vi "NEW数据采集传输系统.vi"() -> ()   [LabVIEW 2016, in "数据传输系统-04.lvlib"]
uses:
  <vilib>/Utility/miscctls.llb/LVPointTypeDef.ctl
  <vilib>/picture/picture.llb/imagedata.ctl
  <vilib>/Utility/config.llb/NI_LVConfig.lvlib
  update/update.lvlib
panel:
  in  "query":bool caption="返回"
  in  "每日自动重发":bool
  out "ADCP流程":string
  out "循环运行次数":i32
  out "上传动作":string
  out "在线ADCP分层数据时间":string
  out "海流计数据时间":string
  out "海流计流程":string
  in  "调试":u16(ring) items=["实时小时数据", "2086上传", "剖面多参数"]
  out "队列数量":u32
  out "数据查询指令":string
  out "2086上传":bool caption="2086"
  out "小时数据发送次数":i32
  out "选择发送的参数":string
  out "数值":i32
  in  "串口透传":bool
  in  "共享MN":bool
  out "剖面数据补发":bool
  out "日志信息补发":bool
  out "数据补发":bool
  in  "自动更新":bool
  in  "数据补传":bool caption="确定"
  out "数据库打开失败次数":dbl
  out "与工控通信指示灯":bool caption="与工控通信"
  out "判断数据反馈":enum16{"非严格判断", "严格判断", "不判断"}(ring)
  in  "暂停上传":bool
  in  "配置表":bool caption="确定"
  in  "updateconfiguration":T1={"主机"="27.154.58.30", "用户"="update", "密码"="std23506", "远程路径"="数据传输系统\\平台数据传输系统.exe", "下载文件名"="平台数据传输系统.exe", "软件版本"=""}
  out "标题显示":string
  in  "更新":bool
  in  "系统编码选择框":string(combo)="地表水质量监测"
  out "数据发送通道":enum16{"TCP", "VISA"}(ring)
  in  "baud rate":u32=9600 caption="波特率"
  in  "VISA resource name":refnum<visa-resource-name> caption="VISA资源名称"
  in  "实时数据发送时间间隔/min":i32=1
  in  "数据组合发送":bool
  in  "2011发送":bool
  out "数据发送协议":enum16{"2005-212协议", "2017-212协议"}(ring)=enum."2017-212协议"
  in  "重发时间":T2(ring)
  in  "重发日期":T3(ring)
  in  "开机启动":bool
  in  "每周自动重发":bool=TRUE
  in  "确定":bool
  in  "返回":bool
  in  "PW":string
  in  "MN":string
  in  "PORT":string
  in  "IP":string
  in  "站点设备":string
  in  "站点名称":string
  out "设置超时时间/min":i32=1
  out "状态信息":T4={"1st Error to Convert "=63, "步骤 "=enum."发送数据", "元素"="实时数据", "TCP服务端掉线计数"=0, "TCP掉线时间节点"="2019/05/08 15:24:17"} {"1st Error to Convert" items=["无错误", "参数错误", "内存已满", "超出区域", "文件结束", "文件已打开", "一般文件IO错误", "未找到文件", "文件权限错误", "磁盘已满", "路径副本", "打开过多文件", "未启用", "未找到资源文件", "无法添加资源", "未找到资源", "未找到图像", "图像内存错误", "画笔不存在", "配置错误类型", "配置未找到解析段", "配置解析错误", "配置内存错误", "错误外部代码格式", "错误外部代码偏移量", "外部代码不存在", "空窗口", "销毁窗口错误", "空菜单", "打印已中止", "错误打印记录", "打印驱动程序错误", "打印时窗口错误", "打印时内存错误", "打印对话框错误", "一般打印错误", "无效设备引用句柄", "设备未找到", "设备参数错误", "设备单位错误", "无法打开设备", "设备调用已中止", "一般错误", "用户已取消", "对象ID过低", "对象ID过高", "对象不在堆中", "未知的堆", "错误DefProc ID", "DefProc不在表格中", "范围外信息", "空方法", "未知信息", "不支持管理器调用", "错误地址", "连接过程中", "连接超时", "连接过程中", "不支持网络属性", "网络错误", "正在使用的地址", "系统缺少内存", "连接已中止", "连接已拒绝", "连接未建立", "连接已建立", "连接已关闭", "初始化错误（交互应用程序管理器）", "错误事件发生", "等待无约束事件发生处理程序", "事件发生队列溢出", "错误路径", "未发出信号量", "未识别类型（交互应用程序管理器）"]}
  out "数据接收超时指示灯":bool caption="数据接收超时"
  out "空闲时间/s":string
  out "系统时间":string
  out "实时小时数据上传":bool caption="实时小时数据"
  out "系统状态改变":bool
  out "软件版本":string
  out "掉线指示":bool
  out "核查数据上传":bool caption="核查数据"
  out "配置信息":T5
  in  "参数配置":bool
  out "反控数据发送":bool caption="反控数据"
  out "读取报文显示":string
  out "发送报文显示":string
  out "心跳包":bool
  out "通信状态":bool
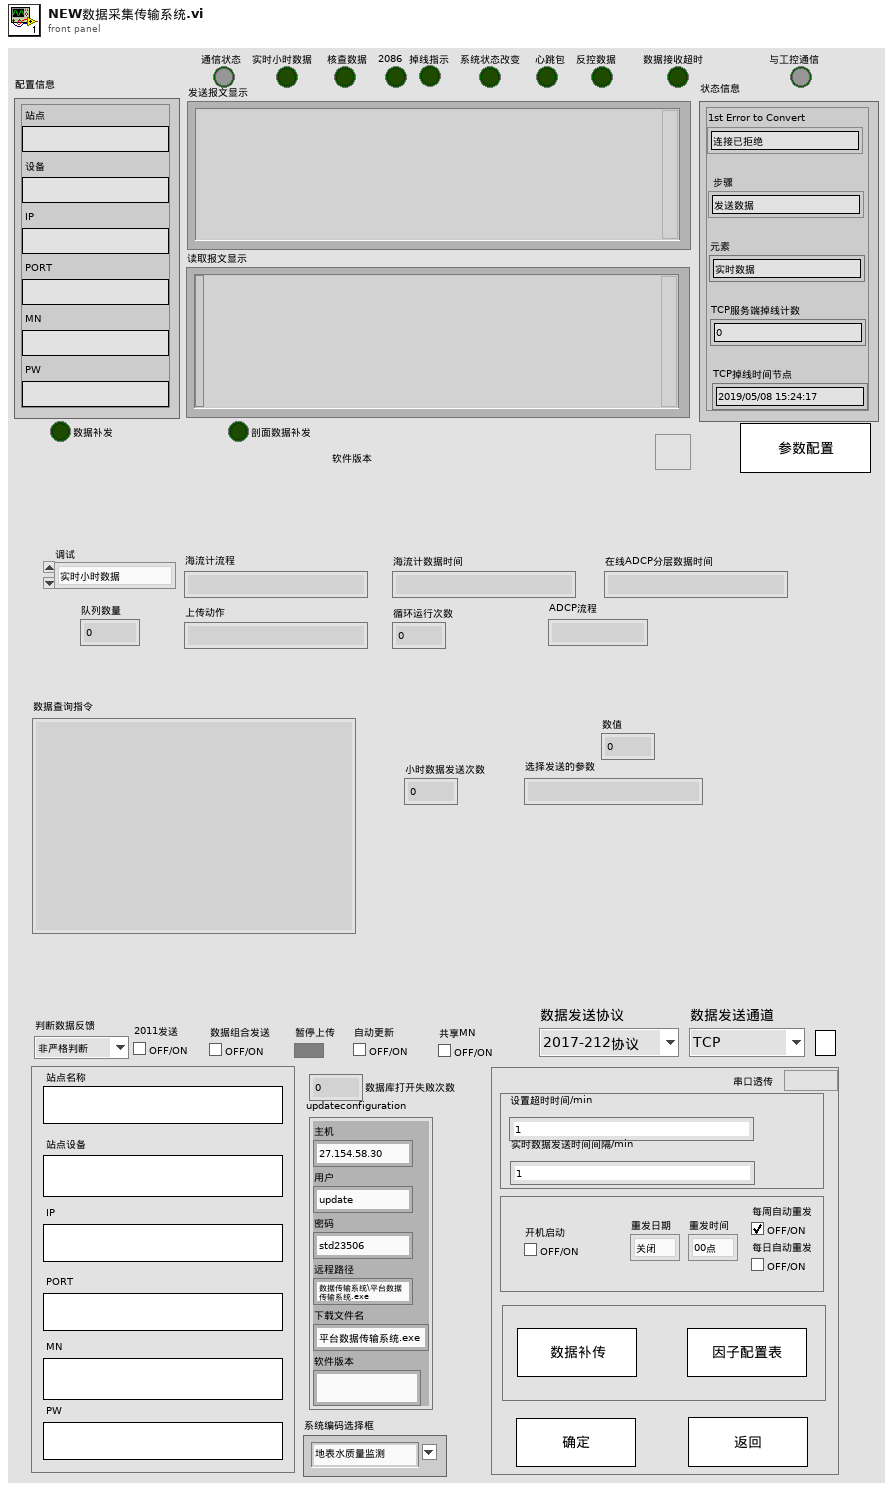
[diagram p1: front panel]
types:
  T1 = cluster{"主机":string, "用户":string, "密码":string, "远程路径":string, "下载文件名":string, "软件版本":string}
  T2 = enum16{"00点", "01点", "02点", "03点", "04点", "05点", "06点", "07点", "08点", "09点", "10点", "11点", "12点", "13点", "14点", "15点", "16点", "17点", "18点", "19点", "20点", "21点", "22点", "23点"}
  T3 = enum16{"关闭", "星期日", "星期一", "星期二", "星期三", "星期四", "星期五", "星期六"}
  T4 = cluster{"1st Error to Convert ":i32, "步骤 ":enum16{"打开连接", "发送数据", "读取数据", "数据处理", "关闭连接"}, "元素":string, "TCP服务端掉线计数":i32, "TCP掉线时间节点":string}
  T5 = cluster{"站点":string, "设备":string, "IP":string, "PORT":string, "MN":string, "PW":string}
  T6 = typedef "imagedata.ctl" = cluster{"image type":i32, "image depth":i32, "image":u8[], "mask":u8[], "colors":u32[], "Rectangle":cluster{"left":i16, "top":i16, "right":i16, "bottom":i16}}
  T7 = typedef "LVPointTypeDef.ctl" = cluster{"Horizontal":i16, "Vertical":i16}
  T8 = cluster{"setini":string, "sysini":string, "hechaini":string, "actualwrite":string, "actualread":string, "datasent":string, "反控命令信息队列":string, "反控与仪器交互":string}
  T9 = cluster{"配置表格[0]":string, "配置表格[1]":string, "配置表格[2]":string, "配置表格[3]":string, "配置表格[4]":string, "配置表格[5]":string, "配置表格[6]":string, "配置表格[7]":string, "配置表格[8]":string, "配置表格[9]":string, "配置表格[10]":string, "配置表格[11]":string, "配置表格[12]":string, "配置表格[13]":string, "配置表格[14]":string, "配置表格[15]":string, "配置表格[16]":string, "配置表格[17]":string, "配置表格[18]":string, "配置表格[19]":string, "配置表格[20]":string, "配置表格[21]":string, "配置表格[22]":string, "配置表格[23]":string, "配置表格[24]":string, "配置表格[25]":string, "配置表格[26]":string, "配置表格[27]":string, "配置表格[28]":string, "配置表格[29]":string, "配置表格[30]":string, "配置表格[31]":string, "配置表格[32]":string, "配置表格[33]":string, "配置表格[34]":string, "配置表格[35]":string, "配置表格[36]":string, "配置表格[37]":string, "配置表格[38]":string, "配置表格[39]":string, "配置表格[40]":string, "配置表格[41]":string, "配置表格[42]":string, "配置表格[43]":string, "配置表格[44]":string, "配置表格[45]":string, "配置表格[46]":string, "配置表格[47]":string, "配置表格[48]":string, "配置表格[49]":string, "配置表格[50]":string, "配置表格[51]":string, "配置表格[52]":string, "配置表格[53]":string, "配置表格[54]":string, "配置表格[55]":string, "配置表格[56]":string, "配置表格[57]":string, "配置表格[58]":string, "配置表格[59]":string, "配置表格[60]":string, "配置表格[61]":string, "配置表格[62]":string, "配置表格[63]":string, "配置表格[64]":string, "配置表格[65]":string, "配置表格[66]":string, "配置表格[67]":string, "配置表格[68]":string, "配置表格[69]":string, "配置表格[70]":string, "配置表格[71]":string, "配置表格[72]":string, "配置表格[73]":string, "配置表格[74]":string, "配置表格[75]":string}
  T10 = cluster{"[0]":dbl, "[1]":dbl, "[2]":dbl, "[3]":dbl, "[4]":dbl, "[5]":dbl, "[6]":dbl, "[7]":dbl, "[8]":dbl, "[9]":dbl, "[10]":dbl, "[11]":dbl, "[12]":dbl, "[13]":dbl, "[14]":dbl, "[15]":dbl, "[16]":dbl, "[17]":dbl, "[18]":dbl, "[19]":dbl, "[20]":dbl, "[21]":dbl, "[22]":dbl, "[23]":dbl, "[24]":dbl, "[25]":dbl, "[26]":dbl, "[27]":dbl, "[28]":dbl, "[29]":dbl, "[30]":dbl, "[31]":dbl, "[32]":dbl, "[33]":dbl, "[34]":dbl, "[35]":dbl, "[36]":dbl, "[37]":dbl, "[38]":dbl, "[39]":dbl, "[40]":dbl, "[41]":dbl, "[42]":dbl, "[43]":dbl, "[44]":dbl, "[45]":dbl, "[46]":dbl, "[47]":dbl, "[48]":dbl, "[49]":dbl, "[50]":dbl, "[51]":dbl, "[52]":dbl, "[53]":dbl, "[54]":dbl, "[55]":dbl, "[56]":dbl, "[57]":dbl, "[58]":dbl, "[59]":dbl, "[60]":dbl, "[61]":dbl, "[62]":dbl, "[63]":dbl, "[64]":dbl, "[65]":dbl, "[66]":dbl, "[67]":dbl, "[68]":dbl, "[69]":dbl, "[70]":dbl, "[71]":dbl, "[72]":dbl, "[73]":dbl, "[74]":dbl, "[75]":dbl}
  T11 = cluster{"时间标识":timestamp, "设备":string, "日志信息":string, "流程参数":string}
  T12 = typedef "NI_LVConfig.lvlib/Config Data RefNum.ctl" = refnum<k1>
  T13 = cluster{"[0]":bool, "[1]":bool, "[2]":bool, "[3]":bool, "[4]":bool, "[5]":bool, "[6]":bool, "[7]":bool, "[8]":bool, "[9]":bool, "[10]":bool, "[11]":bool, "[12]":bool, "[13]":bool, "[14]":bool, "[15]":bool, "[16]":bool, "[17]":bool, "[18]":bool, "[19]":bool, "[20]":bool, "[21]":bool, "[22]":bool, "[23]":bool, "[24]":bool, "[25]":bool, "[26]":bool, "[27]":bool, "[28]":bool, "[29]":bool, "[30]":bool, "[31]":bool, "[32]":bool, "[33]":bool, "[34]":bool, "[35]":bool, "[36]":bool, "[37]":bool, "[38]":bool, "[39]":bool, "[40]":bool, "[41]":bool, "[42]":bool, "[43]":bool, "[44]":bool, "[45]":bool, "[46]":bool, "[47]":bool, "[48]":bool, "[49]":bool, "[50]":bool, "[51]":bool, "[52]":bool, "[53]":bool, "[54]":bool, "[55]":bool, "[56]":bool, "[57]":bool, "[58]":bool, "[59]":bool, "[60]":bool, "[61]":bool, "[62]":bool, "[63]":bool, "[64]":bool, "[65]":bool, "[66]":bool, "[67]":bool, "[68]":bool, "[69]":bool, "[70]":bool, "[71]":bool, "[72]":bool, "[73]":bool, "[74]":bool, "[75]":bool}
  T14 = cluster{"time1":string, "time2":string, "time3":string, "time4":string, "time5":string, "time6":string, "time7":string, "time8":string, "time9":string, "time10":string, "time11":string, "time12":string, "time13":string, "time14":string, "time15":string, "time16":string, "time17":string, "time18":string, "time19":string, "time20":string, "time21":string, "time22":string, "time23":string, "time24":string, "time25":string, "time26":string, "time27":string, "time28":string, "time29":string, "time30":string, "time31":string, "time32":string, "time33":string, "time34":string, "time35":string, "time36":string, "time37":string, "time38":string, "time39":string, "time40":string, "time41":string, "time42":string, "time43":string, "time44":string, "time45":string, "time46":string, "time47":string, "time48":string, "time49":string, "time50":string, "time51":string, "time52":string, "time53":string, "time54":string, "time55":string, "time56":string, "time57":string, "time58":string, "time59":string, "time60":string, "time61":string, "time62":string, "time63":string, "time64":string, "time65":string, "time66":string, "time67":string, "time68":string, "time69":string, "time70":string, "time71":string, "time72":string, "time73":string, "time74":string, "time75":string, "time76":string}
  T15 = cluster{"[0]":string, "[1]":string, "[2]":string, "[3]":string, "[4]":string, "[5]":string, "[6]":string, "[7]":string}
  T16 = cluster{"[0]":string, "[1]":string, "[2]":string, "[3]":string, "[4]":string, "[5]":string, "[6]":string, "[7]":string, "[8]":string, "[9]":string, "[10]":string, "[11]":string, "[12]":string, "[13]":string, "[14]":string}
  T17 = cluster{"[0]":string, "[1]":string, "[2]":string, "[3]":string, "[4]":string, "[5]":string, "[6]":string}
  T18 = cluster{"[0]":string, "[1]":string, "[2]":string, "[3]":string, "[4]":string, "[5]":string, "[6]":string, "[7]":string, "[8]":string, "[9]":string, "[10]":string, "[11]":string, "[12]":string, "[13]":string, "[14]":string, "[15]":string, "[16]":string, "[17]":string}
  T19 = cluster{"[0]":string, "[1]":string, "[2]":string, "[3]":string, "[4]":string, "[5]":string, "[6]":string, "[7]":string, "[8]":string, "[9]":string}
  T20 = cluster{"[0]":string, "[1]":string, "[2]":string, "[3]":string, "[4]":string, "[5]":string, "[6]":string, "[7]":string, "[8]":string, "[9]":string, "[10]":string, "[11]":string, "[12]":string, "[13]":string, "[14]":string, "[15]":string, "[16]":string, "[17]":string, "[18]":string, "[19]":string, "[20]":string, "[21]":string, "[22]":string, "[23]":string, "[24]":string, "[25]":string, "[26]":string, "[27]":string, "[28]":string, "[29]":string, "[30]":string, "[31]":string, "[32]":string, "[33]":string, "[34]":string, "[35]":string, "[36]":string, "[37]":string, "[38]":string, "[39]":string, "[40]":string, "[41]":string, "[42]":string, "[43]":string, "[44]":string, "[45]":string, "[46]":string, "[47]":string, "[48]":string, "[49]":string, "[50]":string, "[51]":string, "[52]":string, "[53]":string, "[54]":string, "[55]":string, "[56]":string, "[57]":string, "[58]":string, "[59]":string, "[60]":string, "[61]":string, "[62]":string, "[63]":string, "[64]":string, "[65]":string, "[66]":string, "[67]":string, "[68]":string, "[69]":string, "[70]":string, "[71]":string, "[72]":string, "[73]":string, "[74]":string, "[75]":string}
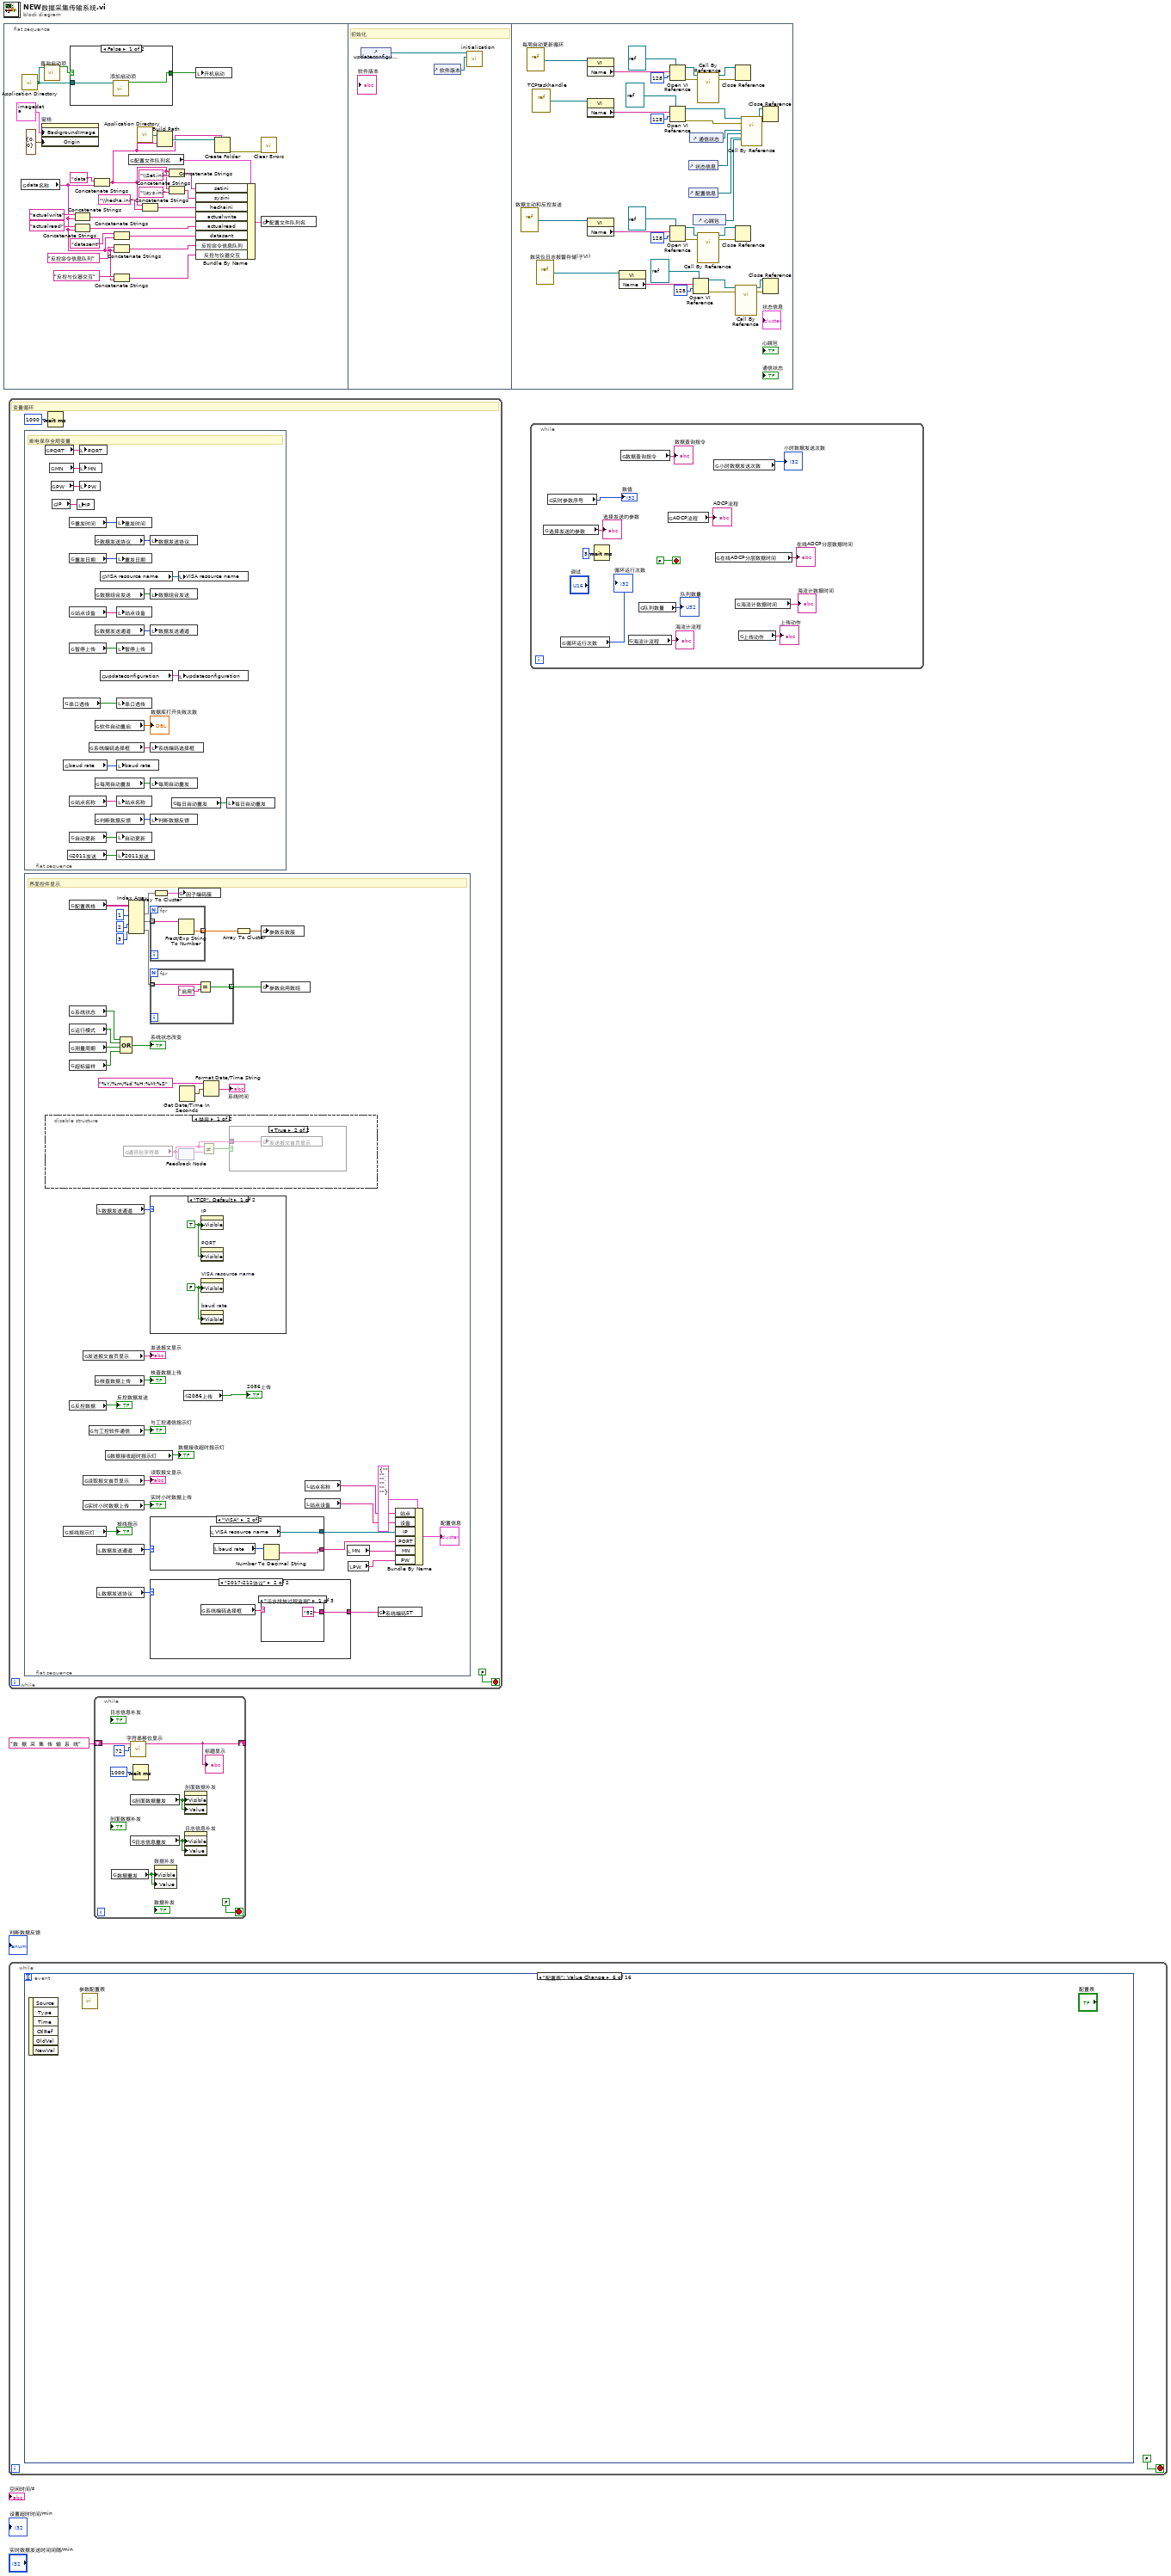
[diagram p0: block diagram]
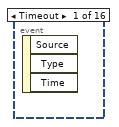
[diagram p2: hidden frame]
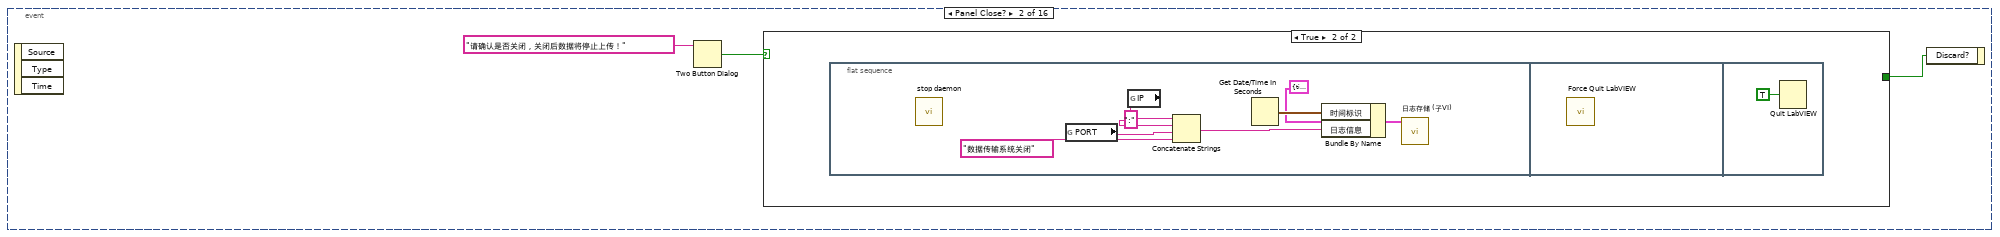
[diagram p3: hidden frame]
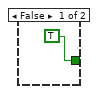
[diagram p4: hidden frame]
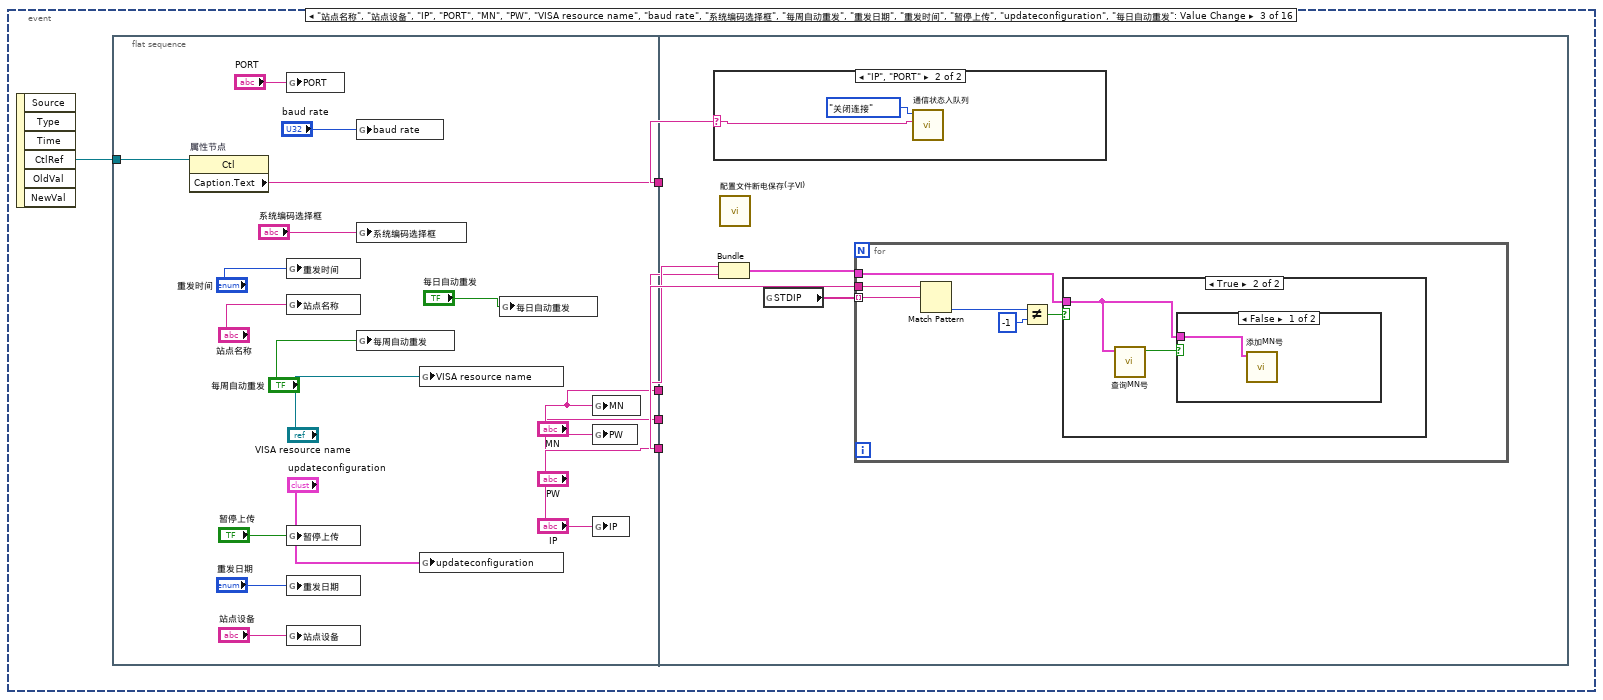
[diagram p5: hidden frame]
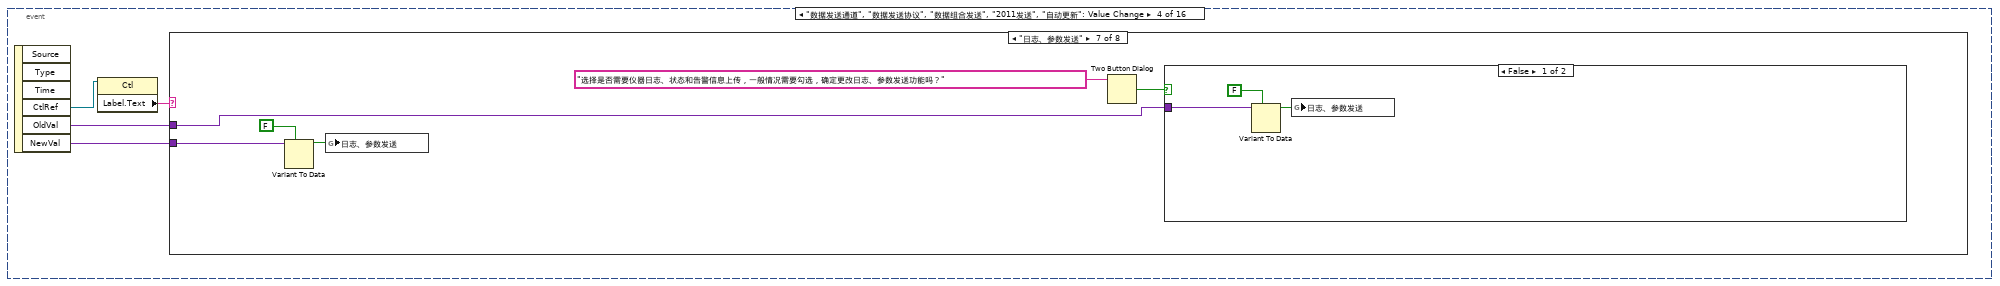
[diagram p9: hidden frame]
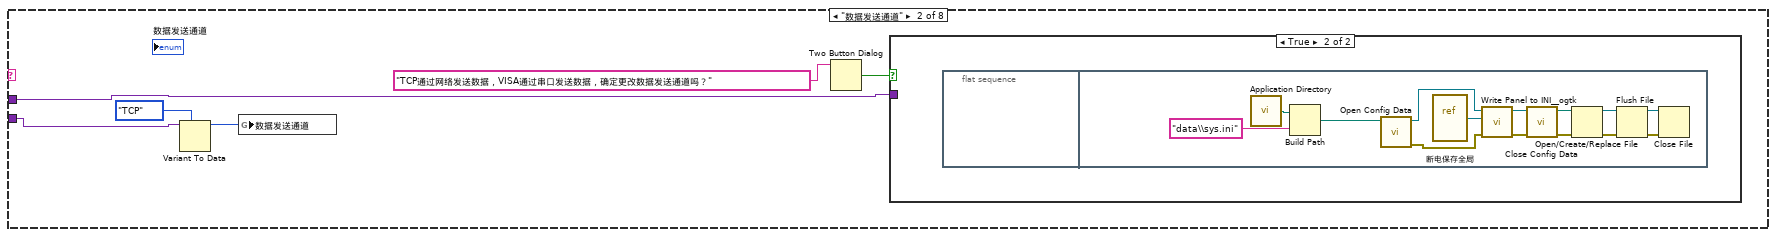
[diagram p11: hidden frame]
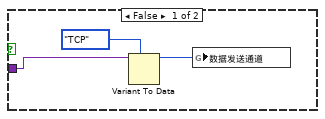
[diagram p12: hidden frame]
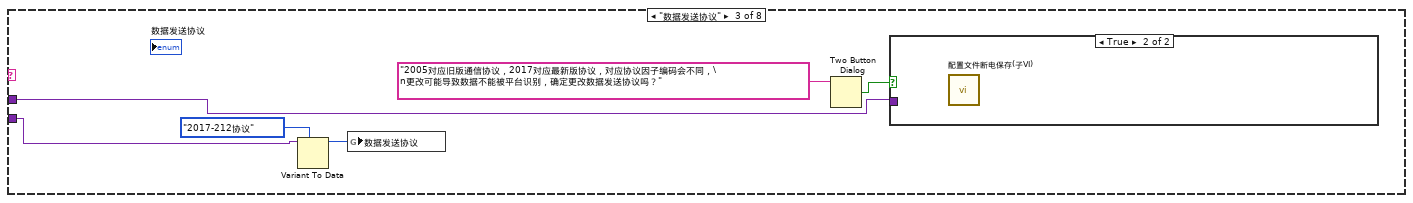
[diagram p13: hidden frame]
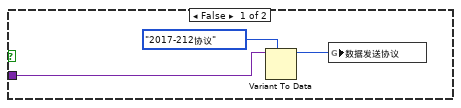
[diagram p14: hidden frame]
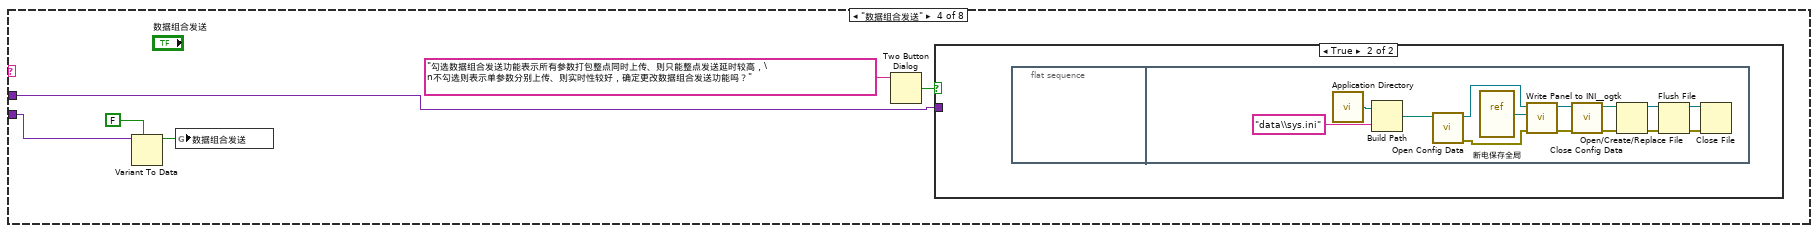
[diagram p15: hidden frame]
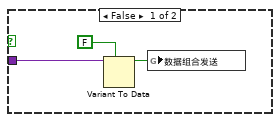
[diagram p16: hidden frame]
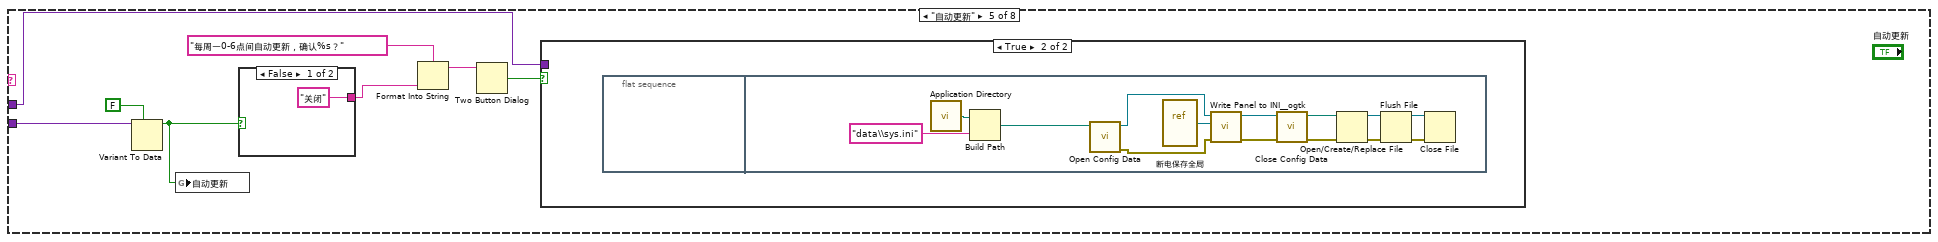
[diagram p17: hidden frame]
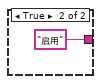
[diagram p18: hidden frame]
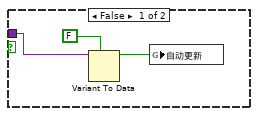
[diagram p19: hidden frame]
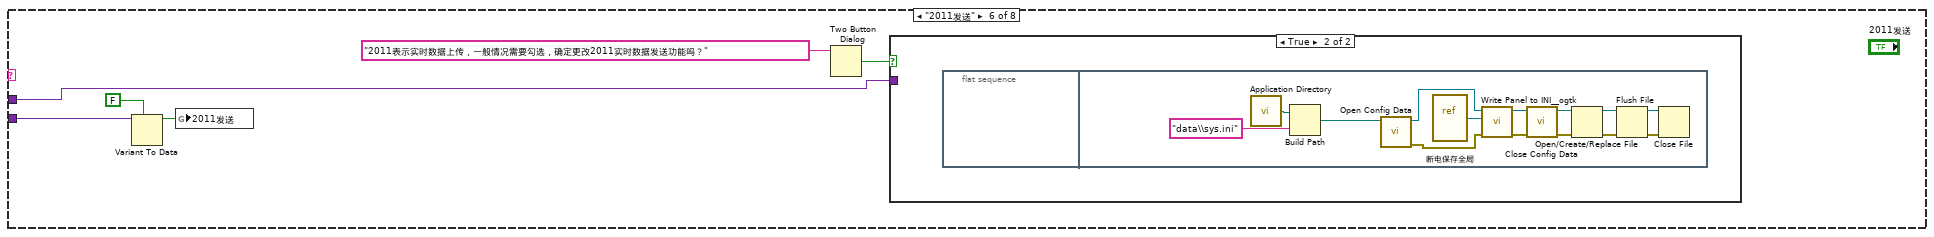
[diagram p20: hidden frame]
diagram:
  n1 = flat-sequence {
    frame #0 {
      n2 = global read "断电保存全局.vi" "data名称"() -> (w3:string)
      n3 = call <vilib>:"Application Directory.vi"() -> ("Application Directory"=w8:path)
      n4 = property on="窗格" class="Pane"("BackgroundImage"=T6 {"image type"=0, "image depth"=24, "image"=array[12288000 elements], "mask"=[], "colors"=[], "Rectangle"={"left"=0, "top"=0, "right"=2560, "bottom"=1600}} ("image data"), "Origin"=T7 {"Horizontal"=0, "Vertical"=0} ("原点")) -> ()  [unwired: 2 in, 2 out]
      n5 = call "查询启动项.vi"("启动文件路径"=w8) -> ("包含启动项"=w7:bool)  [unwired: 9 in, 1 out]
      n6 = case shown="False" w7 {
        selector: w7 -> [_ w33]
        tunnel: w8 -> [w32 _]
        tunnel: [w31 w33] -> w6
        frame False {
          n7 = call "添加启动项.vi"("启动文件路径"=w32) -> ("添加成功标记"=w31:bool)  [unwired: 9 in, 1 out]
        }
        frame True {
        }
      }
      n8 = Concatenate Strings("actualwrite" ("名称（未命名）"), w3) -> (w18:string)
      n9 = Concatenate Strings("actualread" ("名称（未命名）"), w3) -> (w16:string)
      n10 = Concatenate Strings("data" ("对话框窗口（创建文件夹）"), w3) -> (w23:string)
      n11 = Concatenate Strings("datasent" ("名称（未命名）"), w3) -> (w14:string)
      n12 = Concatenate Strings("反控命令信息队列" ("名称（未命名）"), w3) -> (w10:string)
      n13 = Concatenate Strings("反控与仪器交互" ("名称（未命名）"), w3) -> (w11:string)
      n14 = global read "全局1.vi" "配置文件队列名"() -> (w4:T8)
      n15 = call <vilib>:"Application Directory.vi"() -> ("Application Directory"=w29:path)
      n16 = Concatenate Strings(w23, "\\hecha.ini" ("名称或相对路径")) -> (w21:string)
      n17 = Build Path(base path=w29, name or relative path=w23) -> (appended path=w28:path)
      n18 = Concatenate Strings(w23, "\\Set.ini" ("名称或相对路径")) -> (w25:string)
      n19 = Concatenate Strings(w23, "\\sys.ini" ("名称或相对路径")) -> (w22:string)
      n20 = local write "开机启动"(w6) -> ()
      n21 = Bundle By Name(cluster=w4, "setini"=w25, "sysini"=w22, "hechaini"=w21, "actualwrite"=w18, "actualread"=w16, "datasent"=w14, "反控命令信息队列"=w10, "反控与仪器交互"=w11) -> (w2:T8)
      n22 = Create Folder(prompt (Create Folder)=w23, path (use dialog)=w28) -> (error out=w27:errorcluster)  [unwired: 1 in, 2 out]
      n23 = call <vilib>:"Clear Errors.vi"("error in (no error)"=w27) -> ()  [unwired: 5 in, 2 out]
      n24 = global write "全局1.vi" "配置文件队列名"(w2) -> ()
    }
    frame #1 {
      # "初始化"
      n25 = control-ref of="updateconfiguration"() -> (w35:refnum<vi>)
      n26 = control-ref of="软件版本"() -> (w34:refnum<vi>)
      n27 = call "initialization.vi"("软件版本"=w34, "updateconfiguration"=w35) -> ()  [unwired: 9 in]
    }
    frame #2 {
      n28 = vi-ref "数据主动和反控发送.vi"() -> (w36:refnum<vi>)
      n29 = vi-ref "每周自动更新循环.vi"() -> (w56:refnum<vi>)
      n30 = vi-ref "TCPtaskhandle.vi"() -> (w41:refnum<vi>)
      n31 = vi-ref "数采仪日志报警存储(子VI).vi"() -> (w64:refnum<vi>)
      n32 = property class="VI"(reference=w56) -> ("Name"=w49:string)  [unwired: 1 in, 2 out]
      n33 = property class="VI"(reference=w41) -> ("Name"=w48:string)  [unwired: 1 in, 2 out]
      n34 = property class="VI"(reference=w36) -> ("Name"=w63:string)  [unwired: 1 in, 2 out]
      n35 = property class="VI"(reference=w64) -> ("Name"=w71:string)  [unwired: 1 in, 2 out]
      n36 = Open VI Reference(type specifier VI Refnum (for type only)=refnum<vi> refnum, vi path=w49, options=128 ("选项")) -> (vi reference=w51:refnum<vi>, error out=w53:errorcluster)  [unwired: 3 in]
      n37 = Open VI Reference(type specifier VI Refnum (for type only)=refnum<vi> refnum, vi path=w48, options=128 ("选项")) -> (vi reference=w46:refnum<vi>, error out=w44:errorcluster)  [unwired: 3 in]
      n38 = Open VI Reference(type specifier VI Refnum (for type only)=refnum<vi> refnum, vi path=w63, options=128 ("选项")) -> (vi reference=w61:refnum<vi>, error out=w59:errorcluster)  [unwired: 3 in]
      n39 = control-ref of="状态信息"() -> (w39:refnum<vi>)
      n40 = control-ref of="配置信息"() -> (w38:refnum<vi>)
      n41 = control-ref of="通信状态"() -> (w40:refnum<vi>)
      n42 = control-ref of="心跳包"() -> (w37:refnum<vi>)
      n43 = Open VI Reference(type specifier VI Refnum (for type only)=refnum<vi> refnum, vi path=w71, options=128 ("选项")) -> (vi reference=w69:refnum<vi>, error out=w67:errorcluster)  [unwired: 3 in]
      n44 = call-by-ref "?"(reference=w51, error in=w53) -> (reference out=w55:refnum<vi>, error out=w54:errorcluster)  [unwired: 12 in]
      n45 = call-by-ref "?"(reference=w61, error in=w59) -> (reference out=w57:refnum<vi>, error out=w58:errorcluster)  [unwired: 12 in]
      n46 = Close Reference(reference=w55, error in (no error)=w54) -> ()  [unwired: 1 out]
      n47 = Close Reference(reference=w57, error in (no error)=w58) -> ()  [unwired: 1 out]
      n48 = call-by-ref "?"(reference=w69, error in=w67) -> (reference out=w65:refnum<vi>, error out=w66:errorcluster)  [unwired: 12 in]
      n49 = call-by-ref "?"(reference=w46, error in=w44, "心跳包"=w37, "配置信息"=w38, "状态信息"=w39, "通信状态"=w40) -> (reference out=w42:refnum<vi>, error out=w43:errorcluster)  [unwired: 8 in]
      n50 = Close Reference(reference=w42, error in (no error)=w43) -> ()  [unwired: 1 out]
      n51 = Close Reference(reference=w65, error in (no error)=w66) -> ()  [unwired: 1 out]
    }
  }
  n52 = while {
    stop <- FALSE stop-if-true
    # "变量循环"
    n53 = flat-sequence {
      frame #0 {
        # "断电保存全局变量"
        n54 = global read "断电保存全局.vi" "PORT"() -> (w161:string)
        n55 = global read "断电保存全局.vi" "MN"() -> (w160:string)
        n56 = global read "断电保存全局.vi" "PW"() -> (w159:string)
        n57 = global read "断电保存全局.vi" "IP"() -> (w162:string)
        n58 = global read "断电保存全局.vi" "串口透传"() -> (w143:bool)
        n59 = global read "断电保存全局.vi" "baud rate"() -> (w157:u32)
        n60 = global read "断电保存全局.vi" "2011发送"() -> (w153:bool)
        n61 = global read "断电保存全局.vi" "重发时间"() -> (w148:T2)
        n62 = global read "断电保存全局.vi" "重发日期"() -> (w155:T3)
        n63 = global read "断电保存全局.vi" "站点设备"() -> (w163:string)
        n64 = global read "断电保存全局.vi" "暂停上传"() -> (w147:bool)
        n65 = global read "断电保存全局.vi" "站点名称"() -> (w164:string)
        n66 = global read "断电保存全局.vi" "自动更新"() -> (w145:bool)
        n67 = local write "IP"(w162) -> ()
        n68 = local write "PORT"(w161) -> ()
        n69 = local write "MN"(w160) -> ()
        n70 = local write "PW"(w159) -> ()
        n71 = global read "断电保存全局.vi" "系统编码选择框"() -> (w149:string)
        n72 = global read "断电保存全局.vi" "数据发送协议"() -> (w151:enum16{"2005-212协议", "2017-212协议"})
        n73 = global read "断电保存全局.vi" "数据组合发送"() -> (w152:bool)
        n74 = global read "断电保存全局.vi" "数据发送通道"() -> (w150:enum16{"TCP", "VISA"})
        n75 = global read "全局1.vi" "软件自动重启"() -> (→"数据库打开失败次数":dbl)
        n76 = global read "断电保存全局.vi" "每周自动重发"() -> (w156:bool)
        n77 = global read "断电保存全局.vi" "判断数据反馈"() -> (w154:enum16{"非严格判断", "严格判断", "不判断"})
        n78 = global read "断电保存全局.vi" "VISA resource name"() -> (w158:refnum<visa-resource-name>)
        n79 = global read "断电保存全局.vi" "updateconfiguration"() -> (w144:T1)
        n80 = local write "重发时间"(w148) -> ()
        n81 = local write "重发日期"(w155) -> ()
        n82 = local write "站点设备"(w163) -> ()
        n83 = local write "暂停上传"(w147) -> ()
        n84 = local write "串口透传"(w143) -> ()
        n85 = local write "baud rate"(w157) -> ()
        n86 = local write "站点名称"(w164) -> ()
        n87 = local write "自动更新"(w145) -> ()
        n88 = local write "2011发送"(w153) -> ()
        n89 = local write "数据发送协议"(w151) -> ()
        n90 = local write "数据组合发送"(w152) -> ()
        n91 = local write "数据发送通道"(w150) -> ()
        n92 = local write "系统编码选择框"(w149) -> ()
        n93 = local write "每周自动重发"(w156) -> ()
        n94 = local write "判断数据反馈"(w154) -> ()
        n95 = global read "断电保存全局.vi" "每日自动重发"() -> (w142:bool)
        n96 = local write "VISA resource name"(w158) -> ()
        n97 = local write "updateconfiguration"(w144) -> ()
        n98 = local write "每日自动重发"(w142) -> ()
      }
    }
    n99 = flat-sequence {
      frame #0 {
        # "界面控件显示"
        n100 = disable-structure shown="禁用" {
          frame Disabled {
            n101 = global read "全局1.vi" "通讯包字符串"() -> (w115:string)
            n102 = feedback #1(w115) -> (w116:string)
            n103 = feedback-in #1(w115) -> ()
            n104 = Not Equal?(x=w115, y=w116) -> (x != y?=w114:bool)
            n105 = case shown="True" w114 {
              tunnel: w115 -> [_ w117]
              frame False {
              }
              frame True {
                n106 = global write "全局1.vi" "发送报文首页显示"(w117) -> ()
              }
            }
          }
          frame Enabled {
          }
        }
        n107 = global read "全局 数据发送重叠.vi" "掉线指示灯"() -> (→"掉线指示":bool)
        n108 = global read "断电保存全局.vi" "配置表格"() -> (w85:string[][])
        n109 = global read "全局1.vi" "系统状态"() -> (w87:bool)
        n110 = global read "全局1.vi" "运行模式"() -> (w88:bool)
        n111 = global read "全局1.vi" "测量周期"() -> (w89:bool)
        n112 = global read "全局1.vi" "超标留样"() -> (w90:bool)
        n113 = global read "全局1.vi" "反控数据"() -> (→"反控数据发送":bool)
        n114 = global read "全局1.vi" "发送报文首页显示"() -> (→"发送报文显示":string)
        n115 = global read "全局1.vi" "读取报文首页显示"() -> (→"读取报文显示":string)
        n116 = global read "全局1.vi" "实时小时数据上传"() -> (→"实时小时数据上传":bool)
        n117 = global read "全局1.vi" "与工控软件通信"() -> (→"与工控通信指示灯":bool)
        n118 = global read "全局1.vi" "核查数据上传"() -> (→"核查数据上传":bool)
        n119 = local read "数据发送通道"() -> (w95:enum16{"TCP", "VISA"})
        n120 = local read "数据发送通道"() -> (w113:enum16{"TCP", "VISA"})
        n121 = local read "数据发送协议"() -> (w102:enum16{"2005-212协议", "2017-212协议"})
        n122 = global read "全局 数据发送重叠.vi" "数据接收超时指示灯"() -> (→"数据接收超时指示灯":bool)
        n123 = Compound Arithmetic op=OR ("复合运算")(w87, w88, w89, w90) -> (→"系统状态改变":bool)
        n124 = Index Array(array=w85, index (col) #1=1 ("禁用的索引 (列)"), index (col) #2=2 ("索引 (列)"), index (col) #3=3 ("索引 (列)")) -> (element #1=w83:string[], element #2=w77:string[], element #3=w79:string[])  [unwired: 3 in]
        n125 = for {
          tunnel: w77 -> [w119] mode=indexing
          tunnel: [w118] -> w76 mode=indexing
          n126 = Fract/Exp String To Number(string=w119) -> (number=w118:dbl)  [unwired: 3 in, 1 out]
        }
        n127 = for {
          tunnel: w79 -> [w122] mode=indexing
          tunnel: [w120] -> w78 mode=indexing
          n128 = Equal?(x=w122, y="启用") -> (x = y?=w120:bool)
        }
        n129 = case shown="\"TCP\", Default" w95 {
          frame "TCP", Default {
            w123 = TRUE ("可见")
            w124 = FALSE ("可见")
            n130 = property on="IP" class="Str"("Visible"=w123) -> ()  [unwired: 2 in, 2 out]
            n131 = property on="PORT" class="Str"("Visible"=w123) -> ()  [unwired: 2 in, 2 out]
            n132 = property on="VISA resource name" class="VISAName"("Visible"=w124) -> ()  [unwired: 2 in, 2 out]
            n133 = property on="baud rate" class="DigNum (strict)"("Visible"=w124) -> ()  [unwired: 2 in, 2 out]
          }
          frame "VISA" {
            w125 = FALSE ("可见")
            w126 = TRUE ("可见")
            n134 = property on="IP" class="Str"("Visible"=w125) -> ()  [unwired: 2 in, 2 out]
            n135 = property on="PORT" class="Str"("Visible"=w125) -> ()  [unwired: 2 in, 2 out]
            n136 = property on="VISA resource name" class="VISAName"("Visible"=w126) -> ()  [unwired: 2 in, 2 out]
            n137 = property on="baud rate" class="DigNum (strict)"("Visible"=w126) -> ()  [unwired: 2 in, 2 out]
          }
        }
        n138 = case shown="\"VISA\"" w113 {
          tunnel: [w138 w141] -> w110
          tunnel: [w137 w139] -> w107
          frame "TCP", Default {
            n139 = local read "PORT"() -> (w137:string)
            n140 = local read "IP"() -> (w138:string)
          }
          frame "VISA" {
            n141 = local read "VISA resource name"() -> (w141:refnum<visa-resource-name>)
            n142 = local read "baud rate"() -> (w140:u32)
            n143 = Number To Decimal String(number=w140) -> (decimal integer string=w139:string)  [unwired: 1 in]
          }
        }
        n144 = case shown="\"2017-212协议\"" w102 {
          tunnel: [w127 w132] -> w101
          frame "2005-212协议", Default {
            n145 = global read "断电保存全局.vi" "系统编码选择框"() -> (w128:string)
            n146 = case shown="\"地表水体污染源\"" w128 {
              tunnel: ["52" ("设备编码MN") "32" ("设备编码MN") "21" ("设备编码MN")] -> w127
              frame "污水排放过程监测" {
              }
              frame "地表水体污染源" {
              }
              frame "地表水质量监测", Default {
              }
            }
          }
          frame "2017-212协议" {
            n147 = global read "断电保存全局.vi" "系统编码选择框"() -> (w133:string)
            n148 = case shown="\"污水排放过程监测\"" w133 {
              tunnel: ["52" ("设备编码MN") "32" ("设备编码MN") "21" ("设备编码MN")] -> w132
              frame "污水排放过程监测" {
              }
              frame "地表水体污染源" {
              }
              frame "地表水质量监测", Default {
              }
            }
          }
        }
        n149 = Array To Cluster(array=w83) -> (cluster=w86:T9)
        n150 = global write "断电保存全局.vi" "因子编码簇"(w86) -> ()
        n151 = Get Date/Time In Seconds() -> (seconds since 1Jan1904=w103:timestamp)
        n152 = global read "全局1.vi" "2086上传"() -> (→"2086上传":bool)
        n153 = Format Date/Time String(time format string (%c)="%Y/%m/%d %H:%M:%S" ("时间格式字符串(%c)"), seconds (now)=w103) -> (date/time string=→"系统时间":string)  [unwired: 1 in]
        n154 = Array To Cluster(array=w76) -> (cluster=w80:T10)
        n155 = global write "断电保存全局.vi" "参数系数簇"(w80) -> ()
        n156 = global write "断电保存全局.vi" "参数启用数组"(w78) -> ()
        n157 = local read "站点名称"() -> (w109:string)
        n158 = local read "站点设备"() -> (w108:string)
        n159 = local read "MN"() -> (w106:string)
        n160 = local read "PW"() -> (w105:string)
        n161 = global write "全局1.vi" "系统编码ST"(w101) -> ()
        n162 = Bundle By Name(cluster=T5 {"站点"="", "设备"="", "IP"="", "PORT"="", "MN"="", "PW"=""} ("配置信息"), "站点"=w109, "设备"=w108, "IP"=w110, "PORT"=w107, "MN"=w106, "PW"=w105) -> (→"配置信息":T5)
      }
    }
    n163 = Wait (ms)(milliseconds to wait=u32 1000 ("等待时间（毫秒）")) -> ()  [unwired: 1 out]
  }
  n164 = while {
    stop <- FALSE stop-if-true
    n165 = event shown="[5] \"配置表\": Value Change" {
      selector: _ -> [_ _ _ _ _ _ _ _ _ _ _ _ _ _ _ _]
      dyn-events: _ -> [_ _ _ _ _ _ _ _ _ _ _ _ _ _ _ _]
      timeout: _ -> [_ _ _ _ _ _ _ _ _ _ _ _ _ _ _ _]
      event Timeout {
        n166 = event-data() -> ()  [unwired: 1 in, 3 out]
      }
      event Panel Close? {
        n167 = event-data() -> ()  [unwired: 1 in, 3 out]
        n168 = Two Button Dialog(message="请确认是否关闭，关闭后数据将停止上传！" ("消息")) -> (T button?=w167:bool)  [unwired: 2 in]
        n169 = case shown="True" w167 {
          tunnel: [TRUE _] -> w166
          frame False {
          }
          frame True {
            n170 = flat-sequence {
              frame #0 {
                n171 = call "stop daemon.vi"() -> ()  [unwired: 11 in, 1 out]
                n172 = global read "断电保存全局.vi" "PORT"() -> (w173:string)
                n173 = global read "断电保存全局.vi" "IP"() -> (w175:string)
                n174 = Concatenate Strings(w175, ":", w173, "数据传输系统关闭" ("日志信息")) -> (w171:string)
                n175 = Get Date/Time In Seconds() -> (seconds since 1Jan1904=w177:timestamp)
                n176 = Bundle By Name(cluster=T11 {"时间标识"=timestamp(0 s since 1904-01-01), "设备"="数采仪", "日志信息"="", "流程参数"=""} ("data in"), "时间标识"=w177, "日志信息"=w171) -> (w176:T11)
                n177 = call "日志存储 (子VI).vi"("data in"=w176) -> ()  [unwired: 11 in]
              }
              frame #1 {
                n178 = call "Force Quit LabVIEW.vi"() -> ()  [unwired: 10 in, 2 out]
              }
              frame #2 {
                n179 = Quit LabVIEW(quit? (T)=TRUE ("退出？(T)")) -> ()
              }
            }
          }
        }
        n180 = event-data("Discard?"=w166) -> ()  [unwired: 1 in, 1 out]
      }
      event "站点名称", "站点设备", "IP", "PORT", "MN", "PW", "VISA resource name", "baud rate", "系统编码选择框", "每周自动重发", "重发日期", "重发时间", "暂停上传", "updateconfiguration", "每日自动重发": Value Change {
        n181 = event-data() -> ("CtlRef"=w183:refnum<vi>)  [unwired: 1 in, 5 out]
        n182 = flat-sequence {
          tunnel: w183 -> [w185]
          tunnel: [w190] -> w182
          tunnel: ["IP"] -> w181
          tunnel: ["MN"] -> w180
          tunnel: ["PW"] -> w179
          tunnel: w182 -> [w206]
          tunnel: w181 -> [w204]
          tunnel: w180 -> [w203]
          tunnel: w179 -> [w202]
          frame #0 {
            n183 = property on="属性节点" class="Ctl"(reference=w185) -> ("Caption.Text"=w190:string)  [unwired: 1 in, 2 out]
            n184 = global write "断电保存全局.vi" "PORT"("PORT") -> ()
            n185 = global write "断电保存全局.vi" "重发时间"("重发时间") -> ()
            n186 = global write "断电保存全局.vi" "站点名称"("站点名称") -> ()
            n187 = global write "断电保存全局.vi" "暂停上传"("暂停上传") -> ()
            n188 = global write "断电保存全局.vi" "重发日期"("重发日期") -> ()
            n189 = global write "断电保存全局.vi" "站点设备"("站点设备") -> ()
            n190 = global write "断电保存全局.vi" "baud rate"("baud rate") -> ()
            n191 = global write "断电保存全局.vi" "系统编码选择框"("系统编码选择框") -> ()
            n192 = global write "断电保存全局.vi" "每周自动重发"("每周自动重发") -> ()
            n193 = global write "断电保存全局.vi" "VISA resource name"("VISA resource name") -> ()
            n194 = global write "断电保存全局.vi" "updateconfiguration"("updateconfiguration") -> ()
            n195 = global write "断电保存全局.vi" "每日自动重发"("每日自动重发") -> ()
            n196 = global write "断电保存全局.vi" "MN"("MN") -> ()
            n197 = global write "断电保存全局.vi" "PW"("PW") -> ()
            n198 = global write "断电保存全局.vi" "IP"("IP") -> ()
          }
          frame #1 {
            n199 = case shown="\"IP\", \"PORT\"" w206 {
              selector: w206 -> [_ w216]
              frame "假", Default {
              }
              frame "IP", "PORT" {
                n200 = call "通信状态入队列.vi"("发送报文"=w216, "枚举"=enum16{"打开连接", "发送数据", "读取数据", "数据处理", "关闭连接"}."关闭连接") -> ()  [unwired: 9 in, 1 out]
              }
            }
            n201 = Bundle("MN"=w203, "PW"=w202) -> (w201:cluster{"MN":string, "PW":string})  [unwired: 1 in]
            n202 = call "配置文件断电保存(子VI).vi"() -> ()  [unwired: 12 in]
            n203 = global read "断电保存全局.vi" "STDIP"() -> (w205:string[])
            n204 = for {
              tunnel: w205 -> [w212] mode=indexing
              tunnel: w204 -> [w211]
              tunnel: w201 -> [w207]
              n205 = Match Pattern(string=w211, regular expression=w212) -> (offset past match=w210:i32)  [unwired: 1 in, 3 out]
              n206 = Not Equal?(x=w210, y=-1) -> (x != y?=w208:bool)
              n207 = case shown="True" w208 {
                tunnel: w207 -> [_ w214]
                frame False {
                }
                frame True {
                  n208 = call "查询MN号.vi"("簇"=w214) -> ("包含启动项"=w213:bool)  [unwired: 9 in, 1 out]
                  n209 = case shown="False" w213 {
                    tunnel: w214 -> [w215 _]
                    frame False {
                      n210 = call "添加MN号.vi"("簇"=w215) -> ()  [unwired: 9 in, 2 out]
                    }
                    frame True {
                    }
                  }
                }
              }
            }
          }
        }
      }
      event "数据发送通道", "数据发送协议", "数据组合发送", "2011发送", "自动更新": Value Change {
        n211 = event-data() -> ("CtlRef"=w221:refnum<vi>, "OldVal"=w219:variant, "NewVal"=w218:variant)  [unwired: 1 in, 3 out]
        n212 = property class="Ctl"(reference=w221) -> ("Label.Text"=w220:string)  [unwired: 1 in, 2 out]
        n213 = case shown="\"日志、参数发送\"" w220 {
          tunnel: w219 -> [_ w225 w248 w257 w283 w307 w330 w351]
          tunnel: w218 -> [_ w222 w245 w254 w281 w304 w327 w350]
          frame "假", Default {
          }
          frame "数据发送通道" {
            n214 = Variant To Data(type=enum16{"TCP", "VISA"}."TCP" ("数据发送通道"), Variant=w222) -> (data=w223:enum16{"TCP", "VISA"})  [unwired: 1 in, 1 out]
            n215 = global write "断电保存全局.vi" "数据发送通道"(w223) -> ()
            n216 = Two Button Dialog(message="TCP通过网络发送数据，VISA通过串口发送数据，确定更改数据发送通道吗？" ("消息")) -> (T button?=w226:bool)  [unwired: 2 in]
            n217 = case shown="True" w226 {
              tunnel: w225 -> [w229 _]
              frame False {
                n218 = Variant To Data(type=enum16{"TCP", "VISA"}."TCP" ("数据发送通道"), Variant=w229) -> (data=w228:enum16{"TCP", "VISA"})  [unwired: 1 in, 1 out]
                n219 = global write "断电保存全局.vi" "数据发送通道"(w228) -> ()
              }
              frame True {
                n220 = flat-sequence {
                  frame #0 {
                  }
                  frame #1 {
                    n221 = call <vilib>:"Application Directory.vi"() -> ("Application Directory"=w231:path)
                    n222 = Build Path(base path=w231, name or relative path="data\\sys.ini" ("名称或相对路径")) -> (appended path=w233:path)
                    n223 = call <vilib>:"Open Config Data.vi"("configuration file path"=w233) -> ("error out"=w237:errorcluster, "refnum"=w234:T12)  [unwired: 8 in, 1 out]
                    n224 = vi-ref "断电保存全局.vi"() -> (w235:refnum<vi>)
                    n225 = call <userlib>:"Write Panel to INI__ogtk.vi"("error in (no error)"=w237, "VI ref"=w235, "refnum"=w234) -> ("error out"=w238:errorcluster, "refnum out"=w236:T12)  [unwired: 7 in]
                    n226 = call <vilib>:"Close Config Data.vi"("error in (no error)"=w238, "refnum"=w236) -> ("error out"=w243:errorcluster, "file path"=w244:path)  [unwired: 8 in]
                    n227 = Open/Create/Replace File(file path (use dialog)=w244, error in=w243) -> (refnum out=w240:refnum<file>, error out=w239:errorcluster)  [unwired: 4 in, 1 out]
                    n228 = Flush File(refnum=w240, error in=w239) -> (refnum out=w241:refnum<file>, error out=w242:errorcluster)
                    n229 = Close File(refnum=w241, error in=w242) -> ()  [unwired: 2 out]
                  }
                }
              }
            }
          }
          frame "数据发送协议" {
            n230 = Variant To Data(type=enum16{"2005-212协议", "2017-212协议"}."2017-212协议" ("数据"), Variant=w245) -> (data=w246:enum16{"2005-212协议", "2017-212协议"})  [unwired: 1 in, 1 out]
            n231 = global write "断电保存全局.vi" "数据发送协议"(w246) -> ()
            n232 = Two Button Dialog(message="2005对应旧版通信协议，2017对应最新版协议，对应协议因子编码会不同，\n更改可能导致数据不能被平台识别，确定更改数据发送协议吗？" ("消息")) -> (T button?=w249:bool)  [unwired: 2 in]
            n233 = case shown="True" w249 {
              tunnel: w248 -> [w253 _]
              frame False {
                n234 = Variant To Data(type=enum16{"2005-212协议", "2017-212协议"}."2017-212协议" ("数据"), Variant=w253) -> (data=w251:enum16{"2005-212协议", "2017-212协议"})  [unwired: 1 in, 1 out]
                n235 = global write "断电保存全局.vi" "数据发送协议"(w251) -> ()
              }
              frame True {
                n236 = call "配置文件断电保存(子VI).vi"() -> ()  [unwired: 12 in]
              }
            }
          }
          frame "数据组合发送" {
            n237 = Variant To Data(type=FALSE, Variant=w254) -> (data=w255:bool)  [unwired: 1 in, 1 out]
            n238 = global write "断电保存全局.vi" "数据组合发送"(w255) -> ()
            n239 = Two Button Dialog(message="勾选数据组合发送功能表示所有参数打包整点同时上传、则只能整点发送延时较高，\n不勾选则表示单参数分别上传、则实时性较好，确定更改数据组合发送功能吗？" ("消息")) -> (T button?=w258:bool)  [unwired: 2 in]
            n240 = case shown="True" w258 {
              tunnel: w257 -> [w261 _]
              frame False {
                n241 = Variant To Data(type=FALSE, Variant=w261) -> (data=w260:bool)  [unwired: 1 in, 1 out]
                n242 = global write "断电保存全局.vi" "数据组合发送"(w260) -> ()
              }
              frame True {
                n243 = flat-sequence {
                  frame #0 {
                  }
                  frame #1 {
                    n244 = call <vilib>:"Application Directory.vi"() -> ("Application Directory"=w263:path)
                    n245 = Build Path(base path=w263, name or relative path="data\\sys.ini" ("名称或相对路径")) -> (appended path=w265:path)
                    n246 = call <vilib>:"Open Config Data.vi"("configuration file path"=w265) -> ("error out"=w269:errorcluster, "refnum"=w266:T12)  [unwired: 8 in, 1 out]
                    n247 = vi-ref "断电保存全局.vi"() -> (w267:refnum<vi>)
                    n248 = call <userlib>:"Write Panel to INI__ogtk.vi"("error in (no error)"=w269, "VI ref"=w267, "refnum"=w266) -> ("error out"=w270:errorcluster, "refnum out"=w268:T12)  [unwired: 7 in]
                    n249 = call <vilib>:"Close Config Data.vi"("error in (no error)"=w270, "refnum"=w268) -> ("error out"=w275:errorcluster, "file path"=w276:path)  [unwired: 8 in]
                    n250 = Open/Create/Replace File(file path (use dialog)=w276, error in=w275) -> (refnum out=w272:refnum<file>, error out=w271:errorcluster)  [unwired: 4 in, 1 out]
                    n251 = Flush File(refnum=w272, error in=w271) -> (refnum out=w273:refnum<file>, error out=w274:errorcluster)
                    n252 = Close File(refnum=w273, error in=w274) -> ()  [unwired: 2 out]
                  }
                }
              }
            }
          }
          frame "自动更新" {
            n253 = Variant To Data(type=FALSE, Variant=w281) -> (data=w279:bool)  [unwired: 1 in, 1 out]
            n254 = global write "断电保存全局.vi" "自动更新"(w279) -> ()
            n255 = case shown="False" w279 {
              tunnel: ["关闭" "启用"] -> w278
              frame False {
              }
              frame True {
              }
            }
            n256 = Format Into String(format string="每周一0-6点间自动更新，确认%s？" ("消息"), w278) -> (resulting string=w277:string)  [unwired: 2 in, 1 out]
            n257 = Two Button Dialog(message=w277) -> (T button?=w284:bool)  [unwired: 2 in]
            n258 = case shown="True" w284 {
              tunnel: w283 -> [w288 _]
              frame False {
                n259 = Variant To Data(type=FALSE, Variant=w288) -> (data=w287:bool)  [unwired: 1 in, 1 out]
                n260 = global write "断电保存全局.vi" "自动更新"(w287) -> ()
              }
              frame True {
                n261 = flat-sequence {
                  frame #0 {
                  }
                  frame #1 {
                    n262 = call <vilib>:"Application Directory.vi"() -> ("Application Directory"=w290:path)
                    n263 = Build Path(base path=w290, name or relative path="data\\sys.ini" ("名称或相对路径")) -> (appended path=w292:path)
                    n264 = call <vilib>:"Open Config Data.vi"("configuration file path"=w292) -> ("error out"=w296:errorcluster, "refnum"=w293:T12)  [unwired: 8 in, 1 out]
                    n265 = vi-ref "断电保存全局.vi"() -> (w294:refnum<vi>)
                    n266 = call <userlib>:"Write Panel to INI__ogtk.vi"("error in (no error)"=w296, "VI ref"=w294, "refnum"=w293) -> ("error out"=w297:errorcluster, "refnum out"=w295:T12)  [unwired: 7 in]
                    n267 = call <vilib>:"Close Config Data.vi"("error in (no error)"=w297, "refnum"=w295) -> ("error out"=w302:errorcluster, "file path"=w303:path)  [unwired: 8 in]
                    n268 = Open/Create/Replace File(file path (use dialog)=w303, error in=w302) -> (refnum out=w299:refnum<file>, error out=w298:errorcluster)  [unwired: 4 in, 1 out]
                    n269 = Flush File(refnum=w299, error in=w298) -> (refnum out=w300:refnum<file>, error out=w301:errorcluster)
                    n270 = Close File(refnum=w300, error in=w301) -> ()  [unwired: 2 out]
                  }
                }
              }
            }
          }
          frame "2011发送" {
            n271 = Variant To Data(type=FALSE, Variant=w304) -> (data=w305:bool)  [unwired: 1 in, 1 out]
            n272 = global write "断电保存全局.vi" "2011发送"(w305) -> ()
            n273 = Two Button Dialog(message="2011表示实时数据上传，一般情况需要勾选，确定更改2011实时数据发送功能吗？" ("消息")) -> (T button?=w308:bool)  [unwired: 2 in]
            n274 = case shown="True" w308 {
              tunnel: w307 -> [w311 _]
              frame False {
                n275 = Variant To Data(type=FALSE, Variant=w311) -> (data=w310:bool)  [unwired: 1 in, 1 out]
                n276 = global write "断电保存全局.vi" "2011发送"(w310) -> ()
              }
              frame True {
                n277 = flat-sequence {
                  frame #0 {
                  }
                  frame #1 {
                    n278 = call <vilib>:"Application Directory.vi"() -> ("Application Directory"=w313:path)
                    n279 = Build Path(base path=w313, name or relative path="data\\sys.ini" ("名称或相对路径")) -> (appended path=w315:path)
                    n280 = call <vilib>:"Open Config Data.vi"("configuration file path"=w315) -> ("error out"=w319:errorcluster, "refnum"=w316:T12)  [unwired: 8 in, 1 out]
                    n281 = vi-ref "断电保存全局.vi"() -> (w317:refnum<vi>)
                    n282 = call <userlib>:"Write Panel to INI__ogtk.vi"("error in (no error)"=w319, "VI ref"=w317, "refnum"=w316) -> ("error out"=w320:errorcluster, "refnum out"=w318:T12)  [unwired: 7 in]
                    n283 = call <vilib>:"Close Config Data.vi"("error in (no error)"=w320, "refnum"=w318) -> ("error out"=w325:errorcluster, "file path"=w326:path)  [unwired: 8 in]
                    n284 = Open/Create/Replace File(file path (use dialog)=w326, error in=w325) -> (refnum out=w322:refnum<file>, error out=w321:errorcluster)  [unwired: 4 in, 1 out]
                    n285 = Flush File(refnum=w322, error in=w321) -> (refnum out=w323:refnum<file>, error out=w324:errorcluster)
                    n286 = Close File(refnum=w323, error in=w324) -> ()  [unwired: 2 out]
                  }
                }
              }
            }
          }
          frame "日志、参数发送" {
            n287 = Variant To Data(type=FALSE, Variant=w327) -> (data=w328:bool)  [unwired: 1 in, 1 out]
            n288 = global write "断电保存全局.vi" "日志、参数发送"(w328) -> ()
            n289 = Two Button Dialog(message="选择是否需要仪器日志、状态和告警信息上传，一般情况需要勾选，确定更改日志、参数发送功能吗？" ("消息")) -> (T button?=w331:bool)  [unwired: 2 in]
            n290 = case shown="False" w331 {
              tunnel: w330 -> [w334 _]
              frame False {
                n291 = Variant To Data(type=FALSE, Variant=w334) -> (data=w333:bool)  [unwired: 1 in, 1 out]
                n292 = global write "断电保存全局.vi" "日志、参数发送"(w333) -> ()
              }
              frame True {
                n293 = flat-sequence {
                  frame #0 {
                  }
                  frame #1 {
                    n294 = call <vilib>:"Application Directory.vi"() -> ("Application Directory"=w336:path)
                    n295 = Build Path(base path=w336, name or relative path="data\\sys.ini" ("名称或相对路径")) -> (appended path=w338:path)
                    n296 = call <vilib>:"Open Config Data.vi"("configuration file path"=w338) -> ("error out"=w342:errorcluster, "refnum"=w339:T12)  [unwired: 8 in, 1 out]
                    n297 = vi-ref "断电保存全局.vi"() -> (w340:refnum<vi>)
                    n298 = call <userlib>:"Write Panel to INI__ogtk.vi"("error in (no error)"=w342, "VI ref"=w340, "refnum"=w339) -> ("error out"=w343:errorcluster, "refnum out"=w341:T12)  [unwired: 7 in]
                    n299 = call <vilib>:"Close Config Data.vi"("error in (no error)"=w343, "refnum"=w341) -> ("error out"=w348:errorcluster, "file path"=w349:path)  [unwired: 8 in]
                    n300 = Open/Create/Replace File(file path (use dialog)=w349, error in=w348) -> (refnum out=w345:refnum<file>, error out=w344:errorcluster)  [unwired: 4 in, 1 out]
                    n301 = Flush File(refnum=w345, error in=w344) -> (refnum out=w346:refnum<file>, error out=w347:errorcluster)
                    n302 = Close File(refnum=w346, error in=w347) -> ()  [unwired: 2 out]
                  }
                }
              }
            }
          }
          frame "判断数据反馈" {
            n303 = Two Button Dialog(message="判断数据反馈是针对平台能有反馈的情况，\n1.严格判断反馈-收不到反馈一直重发\n2.非严格判断-重发5次后跳过该数据\n3.不判断反馈针对平台没有反馈的情况\n确定更改判断数据反馈功能吗？" ("消息")) -> (T button?=w352:bool)  [unwired: 2 in]
            n304 = case shown="False" w352 {
              tunnel: w351 -> [_ _]
              tunnel: w350 -> [w355 w357]
              frame False {
                n305 = Variant To Data(type=enum16{"非严格判断", "严格判断", "不判断"}."非严格判断" ("判断数据反馈"), Variant=w355) -> (data=w354:enum16{"非严格判断", "严格判断", "不判断"})  [unwired: 1 in, 1 out]
                n306 = local write "判断数据反馈"(w354) -> ()
              }
              frame True {
                n307 = flat-sequence {
                  tunnel: w357 -> [w358]
                  frame #0 {
                    n308 = Variant To Data(type=enum16{"非严格判断", "严格判断", "不判断"}."非严格判断" ("判断数据反馈"), Variant=w358) -> (data=w360:enum16{"非严格判断", "严格判断", "不判断"})  [unwired: 1 in, 1 out]
                    n309 = global write "断电保存全局.vi" "判断数据反馈"(w360) -> ()
                  }
                  frame #1 {
                    n310 = call <vilib>:"Application Directory.vi"() -> ("Application Directory"=w361:path)
                    n311 = Build Path(base path=w361, name or relative path="data\\sys.ini" ("名称或相对路径")) -> (appended path=w363:path)
                    n312 = call <vilib>:"Open Config Data.vi"("configuration file path"=w363) -> ("error out"=w367:errorcluster, "refnum"=w364:T12)  [unwired: 8 in, 1 out]
                    n313 = vi-ref "断电保存全局.vi"() -> (w365:refnum<vi>)
                    n314 = call <userlib>:"Write Panel to INI__ogtk.vi"("error in (no error)"=w367, "VI ref"=w365, "refnum"=w364) -> ("error out"=w368:errorcluster, "refnum out"=w366:T12)  [unwired: 7 in]
                    n315 = call <vilib>:"Close Config Data.vi"("error in (no error)"=w368, "refnum"=w366) -> ("error out"=w373:errorcluster, "file path"=w374:path)  [unwired: 8 in]
                    n316 = Open/Create/Replace File(file path (use dialog)=w374, error in=w373) -> (refnum out=w370:refnum<file>, error out=w369:errorcluster)  [unwired: 4 in, 1 out]
                    n317 = Flush File(refnum=w370, error in=w369) -> (refnum out=w371:refnum<file>, error out=w372:errorcluster)
                    n318 = Close File(refnum=w371, error in=w372) -> ()  [unwired: 2 out]
                  }
                }
              }
            }
          }
        }
      }
      event "确定": Value Change {
        n319 = event-data() -> ()  [unwired: 1 in, 6 out]
        n320 = call "通信状态入队列.vi"("枚举"=enum16{"打开连接", "发送数据", "读取数据", "数据处理", "关闭连接"}."关闭连接") -> ()  [unwired: 10 in, 1 out]
      }
      event "配置表": Value Change {
        n321 = event-data() -> ()  [unwired: 1 in, 6 out]
        n322 = call "参数配置表.vi"() -> ()  [unwired: 12 in]
      }
      event "query": Value Change {
        n323 = event-data() -> ()  [unwired: 1 in, 6 out]
        n324 = call "Query Dig.vi"() -> ()  [unwired: 12 in]
      }
      event "串口透传": Value Change {
        n325 = event-data() -> ()  [unwired: 1 in, 6 out]
        n326 = flat-sequence {
          frame #0 {
            n327 = global write "断电保存全局.vi" "串口透传"("串口透传") -> ()
          }
          frame #1 {
            n328 = call "配置文件断电保存(子VI).vi"() -> ()  [unwired: 12 in]
          }
        }
        n329 = call "串口配置.vi"() -> ()  [unwired: 12 in]
      }
      event "参数配置": Value Change {
        n330 = event-data() -> ()  [unwired: 1 in, 6 out]
        n331 = local read "MN"() -> (w381:string)
        n332 = local read "PW"() -> (w380:string)
        n333 = property on="窗格" class="Pane"("Origin"=T7 {"Horizontal"=0, "Vertical"=1000} ("原点")) -> ()  [unwired: 2 in, 2 out]
        n334 = call <vilib>:"Application Directory.vi"() -> ("Application Directory"=w383:path)
        n335 = Bundle("MN"=w381, "PW"=w380) -> (w379:cluster{"MN":string, "PW":string})  [unwired: 1 in]
        n336 = call "查询启动项.vi"("启动文件路径"=w383) -> ("error out"=w378:errorcluster, "包含启动项"=w382:bool)  [unwired: 9 in]
        n337 = local write "开机启动"(w382) -> ()
        n338 = call "查询MN号.vi"("error in (no error)"=w378, "簇"=w379) -> ("包含启动项"=w377:bool)  [unwired: 8 in, 1 out]
        n339 = local write "共享MN"(w377) -> ()
      }
      event "返回": Value Change {
        n340 = event-data() -> ()  [unwired: 1 in, 6 out]
        n341 = property on="窗格" class="Pane"("Origin"=T7 {"Horizontal"=0, "Vertical"=0} ("原点")) -> ()  [unwired: 2 in, 2 out]
      }
      event "数据补传": Value Change {
        n342 = event-data() -> ()  [unwired: 1 in, 6 out]
        n343 = global read "全局1.vi" "数据发送起始时间"() -> (w388:timestamp)
        n344 = call "数据补传对话框.vi"("起始时间"=w388) -> ("参数数值 2"=w387:T13, "结束时间输出"=w389:timestamp, "起始时间输出"=w390:timestamp, "输出"=w391:bool, "只补小时数据输出"=w386:bool)  [unwired: 6 in]
        n345 = case shown="True" w391 {
          tunnel: w390 -> [_ w401]
          tunnel: w389 -> [_ w402]
          tunnel: w387 -> [_ w398]
          tunnel: w386 -> [_ w400]
          frame False {
            n346 = global write "断电保存全局.vi" "数据重发"(FALSE ("数据重发")) -> ()
          }
          frame True {
            w399 = TRUE ("数据重发")
            n347 = global write "全局1.vi" "数据发送起始时间"(w401) -> ()
            n348 = global write "断电保存全局.vi" "数据重发结束时间"(w402) -> ()
            n349 = Cluster To Array(cluster=w398) -> (array=w396:bool[])
            n350 = global read "全局 水样时间.vi" "水样数据索引"() -> (w397:T14)
            n351 = Format Date/Time String(time format string (%c)="%Y/%m/%d %H:%M:%S" ("时间格式字符串(%c)"), seconds (now)=w401) -> (date/time string=w394:string)  [unwired: 1 in]
            n352 = Cluster To Array(cluster=w397) -> (array=w395:string[])
            n353 = global write "断电保存全局.vi" "数据重发"(w399) -> ()
            n354 = case shown="False" w400 {
              tunnel: w394 -> [w409 _]
              tunnel: w399 -> [w410 _]
              frame False {
                n355 = global write "全局 水样时间.vi" "在线ADCP分层数据时间"(w409) -> ()
                n356 = global write "全局 水样时间.vi" "海流计数据时间"(w409) -> ()
                n357 = global write "断电保存全局.vi" "日志信息重发"(w410) -> ()
                n358 = global write "断电保存全局.vi" "剖面数据重发"(w410) -> ()
                n359 = global write "全局 水样时间.vi" "剖面多参数数据时间"(w409) -> ()
                n360 = global write "全局 水样时间.vi" "剖面数据时间"(w409) -> ()
                n361 = global write "断电保存全局.vi" "数据重发时间戳"(w409) -> ()
                n362 = Initialize Array(w409, 8 ("维数大小")) -> (w413:string[])
                n363 = Initialize Array(w409, 15 ("维数大小")) -> (w414:string[])
                n364 = Array To Cluster(array=w413) -> (cluster=w412:T15)
                n365 = global read "断电保存全局.vi" "数据组合发送"() -> (w417:bool)
                n366 = global write "全局 时间2.vi" "仪器日志索引"(w412) -> ()
                n367 = Array To Cluster(array=w414) -> (cluster=w415:T16)
                n368 = case shown="False" w417 {
                  tunnel: w409 -> [w418 _]
                  frame False {
                    n369 = global write "全局 时间2.vi" "标样核查索引起始时间"(w418) -> ()
                    n370 = global write "全局 时间2.vi" "加标回收索引起始时间"(w418) -> ()
                    n371 = global write "全局 时间2.vi" "跨度核查索引起始时间"(w418) -> ()
                    n372 = global write "全局 时间2.vi" "3092日志索引起始时间"(w418) -> ()
                    n373 = global write "全局 时间2.vi" "零点核查索引起始时间"(w418) -> ()
                    n374 = Initialize Array(w418, 7 ("维数大小")) -> (w422:string[])
                    n375 = Initialize Array(w418, 8 ("维数大小")) -> (w421:string[])
                    n376 = Initialize Array(w418, 18 ("维数大小")) -> (w425:string[])
                    n377 = Initialize Array(w418, 10 ("维数大小")) -> (w430:string[])
                    n378 = Array To Cluster(array=w421) -> (cluster=w420:T15)
                    n379 = Array To Cluster(array=w422) -> (cluster=w423:T17)
                    n380 = global write "全局 时间2.vi" "平行样索引"(w423) -> ()
                    n381 = global write "全局 时间2.vi" "加标回收索引"(w423) -> ()
                    n382 = global write "全局 时间2.vi" "仪器日志索引"(w420) -> ()
                    n383 = Array To Cluster(array=w425) -> (cluster=w426:T18)
                    n384 = Array To Cluster(array=w430) -> (cluster=w429:T19)
                    n385 = global write "全局 时间2.vi" "标样核查索引"(w426) -> ()
                    n386 = global write "全局 时间2.vi" "集成干预索引"(w426) -> ()
                    n387 = global write "全局 时间2.vi" "跨度核查索引"(w429) -> ()
                    n388 = global write "全局 时间2.vi" "零点核查索引"(w429) -> ()
                  }
                  frame True {
                  }
                }
                n389 = global write "全局 时间2.vi" "仪器参数索引"(w415) -> ()
              }
              frame True {
                n390 = global write "断电保存全局.vi" "2011发送"(FALSE ("2011发送")) -> ()
              }
            }
            n391 = for {
              tunnel: w396 -> [w408] mode=indexing
              tunnel: w395 -> [w406] mode=indexing
              tunnel: w394 -> [w407]
              tunnel: [w405] -> w393 mode=indexing
              n392 = Select(t=w407, s=w408, f=w406) -> (s? t:f=w405:string)
            }
            n393 = Array To Cluster(array=w393) -> (cluster=w403:T20)
            n394 = global write "全局 水样时间.vi" "水样数据索引"(w403) -> ()
          }
        }
      }
      event "调试": Value Change {
        n395 = event-data() -> ("CtlRef"=w436:refnum<vi>)  [unwired: 1 in, 3 out]
        n396 = global read "全局1.vi" "配置文件队列名"() -> (w443:T8)
        n397 = property class="Ring (strict)"(reference=w436) -> ("Value"=w435:u16)  [unwired: 1 in, 2 out]
        n398 = Unbundle By Name(w443) -> ("datasent"=w442:string)
        n399 = property on="调试" class="Ring (strict)"() -> ("Strings []"=w440:string[])  [unwired: 2 in, 2 out]
        n400 = Index Array(array=w440, index=w435) -> (element=w437:string)
        n401 = Obtain Queue(name (unnamed)=w442, element data type="", create if not found? (T)=TRUE ("如未找到则创建？(T)")) -> (queue out=w439:refnum<queue>, error out=w438:errorcluster)  [unwired: 2 in, 1 out]
        n402 = Enqueue Element(queue=w439, element=w437, error in (no error)=w438) -> (queue out=w433:refnum<queue>, error out=w432:errorcluster)  [unwired: 1 in, 1 out]
        n403 = Release Queue(queue=w433, error in (no error)=w432) -> ()  [unwired: 1 in, 3 out]
      }
      event "开机启动": Value Change {
        n404 = event-data() -> ("CtlRef"=w445:refnum<vi>, "OldVal"=w444:bool, "NewVal"=w446:bool)  [unwired: 1 in, 3 out]
        n405 = case shown="False" w446 {
          tunnel: w445 -> [w448 w461]
          tunnel: w444 -> [w447 w460]
          frame False {
            n406 = Two Button Dialog(message="是否删除开机启动？" ("消息"), 1:"否" ("F按钮名称（“取消”）"), 2:"是" ("T按钮名称（“确定”）")) -> (T button?=w449:bool)
            n407 = case shown="True" w449 {
              tunnel: w448 -> [w454 _]
              tunnel: w447 -> [w453 _]
              frame False {
                n408 = property class="Bool (strict)"(reference=w454, "Value"=w453) -> ()  [unwired: 1 in, 2 out]
              }
              frame True {
                n409 = call <vilib>:"Application Directory.vi"() -> ("Application Directory"=w456:path)
                n410 = call "删除启动项.vi"("启动文件路径"=w456) -> ("删除标记"=w455:bool)  [unwired: 9 in, 1 out]
                n411 = case shown="True" w455 {
                  tunnel: ["删除开机启动失败" ("T按钮名称（“确定”）") "删除开机启动成功" ("T按钮名称（“确定”）")] -> w457
                  frame False {
                  }
                  frame True {
                  }
                }
                n412 = One Button Dialog(message=w457) -> ()  [unwired: 1 in, 1 out]
              }
            }
          }
          frame True {
            n413 = Two Button Dialog(message="是否添加开机启动？" ("消息"), 1:"否" ("F按钮名称（“取消”）"), 2:"是" ("T按钮名称（“确定”）")) -> (T button?=w462:bool)
            n414 = case shown="True" w462 {
              tunnel: w461 -> [w467 _]
              tunnel: w460 -> [w466 _]
              frame False {
                n415 = property class="Bool (strict)"(reference=w467, "Value"=w466) -> ()  [unwired: 1 in, 2 out]
              }
              frame True {
                n416 = call <vilib>:"Application Directory.vi"() -> ("Application Directory"=w470:path)
                n417 = call "添加启动项.vi"("启动文件路径"=w470) -> ("添加成功标记"=w469:bool)  [unwired: 9 in, 1 out]
                n418 = case shown="True" w469 {
                  tunnel: ["添加开机启动失败" ("T按钮名称（“确定”）") "添加开机启动成功" ("T按钮名称（“确定”）")] -> w468
                  frame False {
                  }
                  frame True {
                  }
                }
                n419 = One Button Dialog(message=w468) -> ()  [unwired: 1 in, 1 out]
              }
            }
          }
        }
      }
      event "共享MN": Value Change {
        n420 = event-data() -> ("CtlRef"=w474:refnum<vi>, "OldVal"=w473:bool, "NewVal"=w475:bool)  [unwired: 1 in, 3 out]
        n421 = case shown="True" w475 {
          tunnel: w474 -> [w477 w492]
          tunnel: w473 -> [w476 w491]
          frame False {
            n422 = Two Button Dialog(message="是否取消该MN号共享？" ("消息"), 1:"否" ("F按钮名称（“取消”）"), 2:"是" ("T按钮名称（“确定”）")) -> (T button?=w478:bool)
            n423 = case shown="True" w478 {
              tunnel: w477 -> [w483 _]
              tunnel: w476 -> [w482 _]
              frame False {
                n424 = property class="Bool (strict)"(reference=w483, "Value"=w482) -> ()  [unwired: 1 in, 2 out]
              }
              frame True {
                n425 = local read "MN"() -> (w487:string)
                n426 = local read "PW"() -> (w486:string)
                n427 = Bundle("MN"=w487, "PW"=w486) -> (w485:cluster{"MN":string, "PW":string})  [unwired: 1 in]
                n428 = call "删除MN号.vi"("簇"=w485) -> ("删除标记"=w484:bool)  [unwired: 9 in, 1 out]
                n429 = case shown="True" w484 {
                  tunnel: ["取消该MN号共享失败" ("T按钮名称（“确定”）") "取消该MN号共享成功" ("T按钮名称（“确定”）")] -> w488
                  frame False {
                  }
                  frame True {
                  }
                }
                n430 = One Button Dialog(message=w488) -> ()  [unwired: 1 in, 1 out]
              }
            }
          }
          frame True {
            n431 = Two Button Dialog(message="是否添加该MN号共享？" ("消息"), 1:"否" ("F按钮名称（“取消”）"), 2:"是" ("T按钮名称（“确定”）")) -> (T button?=w493:bool)
            n432 = case shown="True" w493 {
              tunnel: w492 -> [w498 _]
              tunnel: w491 -> [w497 _]
              frame False {
                n433 = property class="Bool (strict)"(reference=w498, "Value"=w497) -> ()  [unwired: 1 in, 2 out]
              }
              frame True {
                n434 = local read "MN"() -> (w502:string)
                n435 = local read "PW"() -> (w501:string)
                n436 = Bundle("MN"=w502, "PW"=w501) -> (w500:cluster{"MN":string, "PW":string})  [unwired: 1 in]
                n437 = call "添加MN号.vi"("簇"=w500) -> ("添加成功标记"=w499:bool)  [unwired: 9 in, 1 out]
                n438 = case shown="False" w499 {
                  tunnel: ["添加该MN号共享失败" ("T按钮名称（“确定”）") "添加该MN号共享成功" ("T按钮名称（“确定”）")] -> w503
                  frame False {
                  }
                  frame True {
                  }
                }
                n439 = One Button Dialog(message=w503) -> ()  [unwired: 1 in, 1 out]
              }
            }
          }
        }
      }
      event "更新": Value Change {
        n440 = event-data() -> ()  [unwired: 1 in, 6 out]
        n441 = call "自定义双按钮对话框.vi"("消息"="选择是否从服务器获取最新版本信息？") -> ("正式版/测试版输出"=w506:bool, "输出"=w507:bool)  [unwired: 9 in]
        n442 = case shown="True" w507 {
          tunnel: w506 -> [_ w511]
          frame False {
          }
          frame True {
            # "获取最新版本"
            n443 = local read "updateconfiguration"() -> (w516:T1)
            n444 = Unbundle By Name(w516) -> ("远程路径"=w510:string)
            n445 = case shown="True" w511 {
              tunnel: w510 -> [w517 w518]
              tunnel: [w517 w519] -> w514
              frame False {
                # "正式版"
              }
              frame True {
                # "测试版"
                n446 = String To Path(string=w518) -> (path=w520:path)
                n447 = Strip Path(path=w520) -> (name=w523:string)  [unwired: 1 out]
                n448 = Search and Replace String(input string=w518, search string=w523, replace string="beta/" ("字符串")) -> (result string=w522:string)  [unwired: 5 in, 3 out]
                n449 = Concatenate Strings(w522, w523) -> (w519:string)
              }
            }
            n450 = Search and Replace String(replace all?=TRUE ("替换全部？(F)"), input string=w514, search string="\\" ("替换字符串(\"\")"), replace string="/" ("分隔符(Tab)")) -> (result string=w509:string)  [unwired: 4 in, 3 out]
            n451 = call "Updateinter.vi"("更新包远端地址"=w509, "测试版？"=w511) -> ()  [unwired: 10 in]
          }
        }
      }
      event "IP", "PORT": Mouse Down {
        n452 = event-data() -> ("CtlRef"=w532:refnum<vi>)  [unwired: 1 in, 7 out]
        n453 = property class="Str"(reference=w532) -> (reference out=w530:refnum<vi>, "Value"=w531:string)  [unwired: 1 in, 1 out]
        n454 = call "IP键盘.vi"("OldNumber"=w531) -> ("NewNumber"=w527:string)
        n455 = String Length(string=w527) -> (length=w529:i32)
        n456 = Less Or Equal?(x=w529, y=50) -> (x <= y?=w526:bool)
        n457 = case shown="False" w526 {
          tunnel: w530 -> [w533 w537]
          tunnel: w527 -> [_ w536]
          tunnel: [w533 w537] -> w525
          tunnel: ["127.0.0.1" w536] -> w524
          frame False {
            n458 = One Button Dialog(message="超过ipv4最大长度限制,请重新输入!" ("消息")) -> ()  [unwired: 1 in, 1 out]
          }
          frame True {
          }
        }
        n459 = property class="Str"(reference=w525, "Val(Sgnl)"=w524) -> ()  [unwired: 1 in, 2 out]
      }
    }
  }
  n460 = while {
    shift-right: [w542] -> _
    shift-left: "数  据  采  集  传  输  系  统" ("标题显示") -> [w543]
    stop <- FALSE stop-if-true
    n461 = global read "断电保存全局.vi" "数据重发"() -> (w540:bool)
    n462 = global read "断电保存全局.vi" "剖面数据重发"() -> (w538:bool)
    n463 = global read "断电保存全局.vi" "日志信息重发"() -> (w539:bool)
    n464 = call "字符串移位显示.vi"("字符框大小"=72, "字符串输入"=w543) -> ("移位后字符串"=w542:string)  [unwired: 8 in, 1 out]
    "标题显示" <- w542
    n465 = Wait (ms)(milliseconds to wait=u32 1000 ("等待时间（毫秒）")) -> ()  [unwired: 1 out]
    n466 = property on="数据补发" class="Bool (strict)"("Visible"=w540, "Value"=w540) -> ()  [unwired: 2 in, 2 out]
    n467 = property on="剖面数据补发" class="Bool (strict)"("Visible"=w538, "Value"=w538) -> ()  [unwired: 2 in, 2 out]
    n468 = property on="日志信息补发" class="Bool (strict)"("Visible"=w539, "Value"=w539) -> ()  [unwired: 2 in, 2 out]
  }
  n469 = while {
    stop <- FALSE stop-if-true
    n470 = global read "全局 水样时间.vi" "选择发送的参数"() -> (→"选择发送的参数":string)
    n471 = global read "断电保存全局.vi" "实时参数序号"() -> (→"数值":i32)
    n472 = global read "全局 水样时间.vi" "循环运行次数"() -> (→"循环运行次数":i32)
    n473 = Wait (ms)(milliseconds to wait=u32 5 ("等待时间（毫秒）")) -> ()  [unwired: 1 out]
    n474 = global read "全局 水样时间.vi" "数据查询指令"() -> (→"数据查询指令":string)
    n475 = global read "全局 水样时间.vi" "海流计流程"() -> (→"海流计流程":string)
    n476 = global read "全局 水样时间.vi" "队列数量"() -> (→"队列数量":u32)
    n477 = global read "全局 水样时间.vi" "ADCP流程"() -> (→"ADCP流程":string)
    n478 = global read "全局 小时数据发送次数.vi" "小时数据发送次数"() -> (→"小时数据发送次数":i32)
    n479 = global read "全局 水样时间.vi" "在线ADCP分层数据时间"() -> (→"在线ADCP分层数据时间":string)
    n480 = global read "全局 水样时间.vi" "海流计数据时间"() -> (→"海流计数据时间":string)
    n481 = global read "全局 水样时间.vi" "上传动作"() -> (→"上传动作":string)
  }
